vi "TLB Native Dynamic Events ver 0.16.vi"() -> ()   [LabVIEW 2018]
uses:
  Labview Training Phase 2/Enum Controls/States for Action Engine.ctl
  TLB Type Definitions/State Type Definitions.ctl
  TLB Type Definitions/Intruction Type Definitions.ctl
  TLB Type Definitions/Encoder cluster.ctl
  TLB Type Definitions/PING CLUSTER.ctl
  <vilib>/Studica/Studica Toolkit/NavX/NavX.lvlib
  <vilib>/Studica/Studica Toolkit/Background/DIO Channel.ctl
  Underlying VI's/NavX VI/navX type def.ctl
  <vilib>/myRIO/Instrument Drivers/Utilities/Utilities.lvlib
  <vilib>/Studica/Studica Toolkit/Background/I2C Channel.ctl
  TLB Type Definitions/Vision cluster.ctl
  <vilib>/NI_Real-Time Target Support.lvlib
  TLB Type Definitions/Stepper cluster.ctl
  Experimental VI's/Archived VI's/MOTOR CONTROL NO PID Type Def.ctl
  Underlying VI's/I2C Master VI/I2C MASTER Type Def.ctl
  Underlying VI's/I2C Master VI/I2C_MASTER_WRITE_NEW Type Def.ctl
  <vilib>/userdefined/High Color/IMAQdx.ctl
  Underlying VI's/I2C Master VI/Arduino_Interfacing.ctl
  TLB Type Definitions/Yaw Cluster.ctl
  TLB Type Definitions/Time cluster.ctl
  TLB Type Definitions/Y Stepper cluster.ctl
  Underlying VI's/Modified webcam FGV/Webcam AE.ctl
  Underlying VI's/Elasped Timer/Elapsed timer control.ctl
  Underlying VI's/Motor Control VI with PID/MOTOR CONTROL WITH PID AE DATA MODE TYPE DEF.ctl
  Underlying VI's/Motor Control VI with PID/MOTOR CONTROL WITH PID AE DIRECTION TYPE DEF.ctl
  <vilib>/Utility/RT CPU Load.ctl
panel:
  out "Speed & distance":T1
  out "Object Center Coordinates":cluster{"x":sgl, "y":sgl}
  out "Object detection cluster":T2
  out "Time up flag":bool
  out "Task selection":u8
  in  "Object recognition mode":enum16{"Ball", "Soap", "Gel", "Pipe", "None"}(ring)
  out "NavX Readings":T3
  out "Arduino Data":T4
  out "CPU loads":T5[](array[typedef]) {"ISR (%)" format="%#.2f"; "Idle (%)" format="%#.2f"; "Background (%)" format="%#.2f"; "Normal (%)" format="%#.2f"; "Above Normal (%)" format="%#.2f"; "High (%)" format="%#.2g"; "Timed Structures (%)" format="%#.2g"; "Time Critical (%)" format="%#.2g"; "Total (%)" format="%#.2g"}
  out "TASK ENABLE":bool
  out "Rising Edge":bool
  in  "Green LED":bool
  out "Obstacle detected":bool
  out "I2C Error":errorcluster
  out "State Logic":T6=enum."Startup"
  out "elements":T7[](array[typedef])
  in  "STOP TASK":bool
  in  "OK Button":bool
  in  "STOP":bool
  out "error out":errorcluster
  out "Action Queue Items":i32
  out "State Logic Queue Items":i32
  out "Action Queues items":string[](array[string])=["Hardware reset", "Software reset", ""]
  out "Action State":string
  # "System Health Status Update"
  # "VISION"
  # "TLB FRAMEWORK STATUS"
  # "Test Programme written by Calvin Loke    Dated: 28 Aug 2019\nTest Programme revised by Dr Alex See   Dated 30 Aug 2019\n\nRevision date: 20/03/2020\nProgramme version:   TLB Native Dynamic Events ver 0.14a"
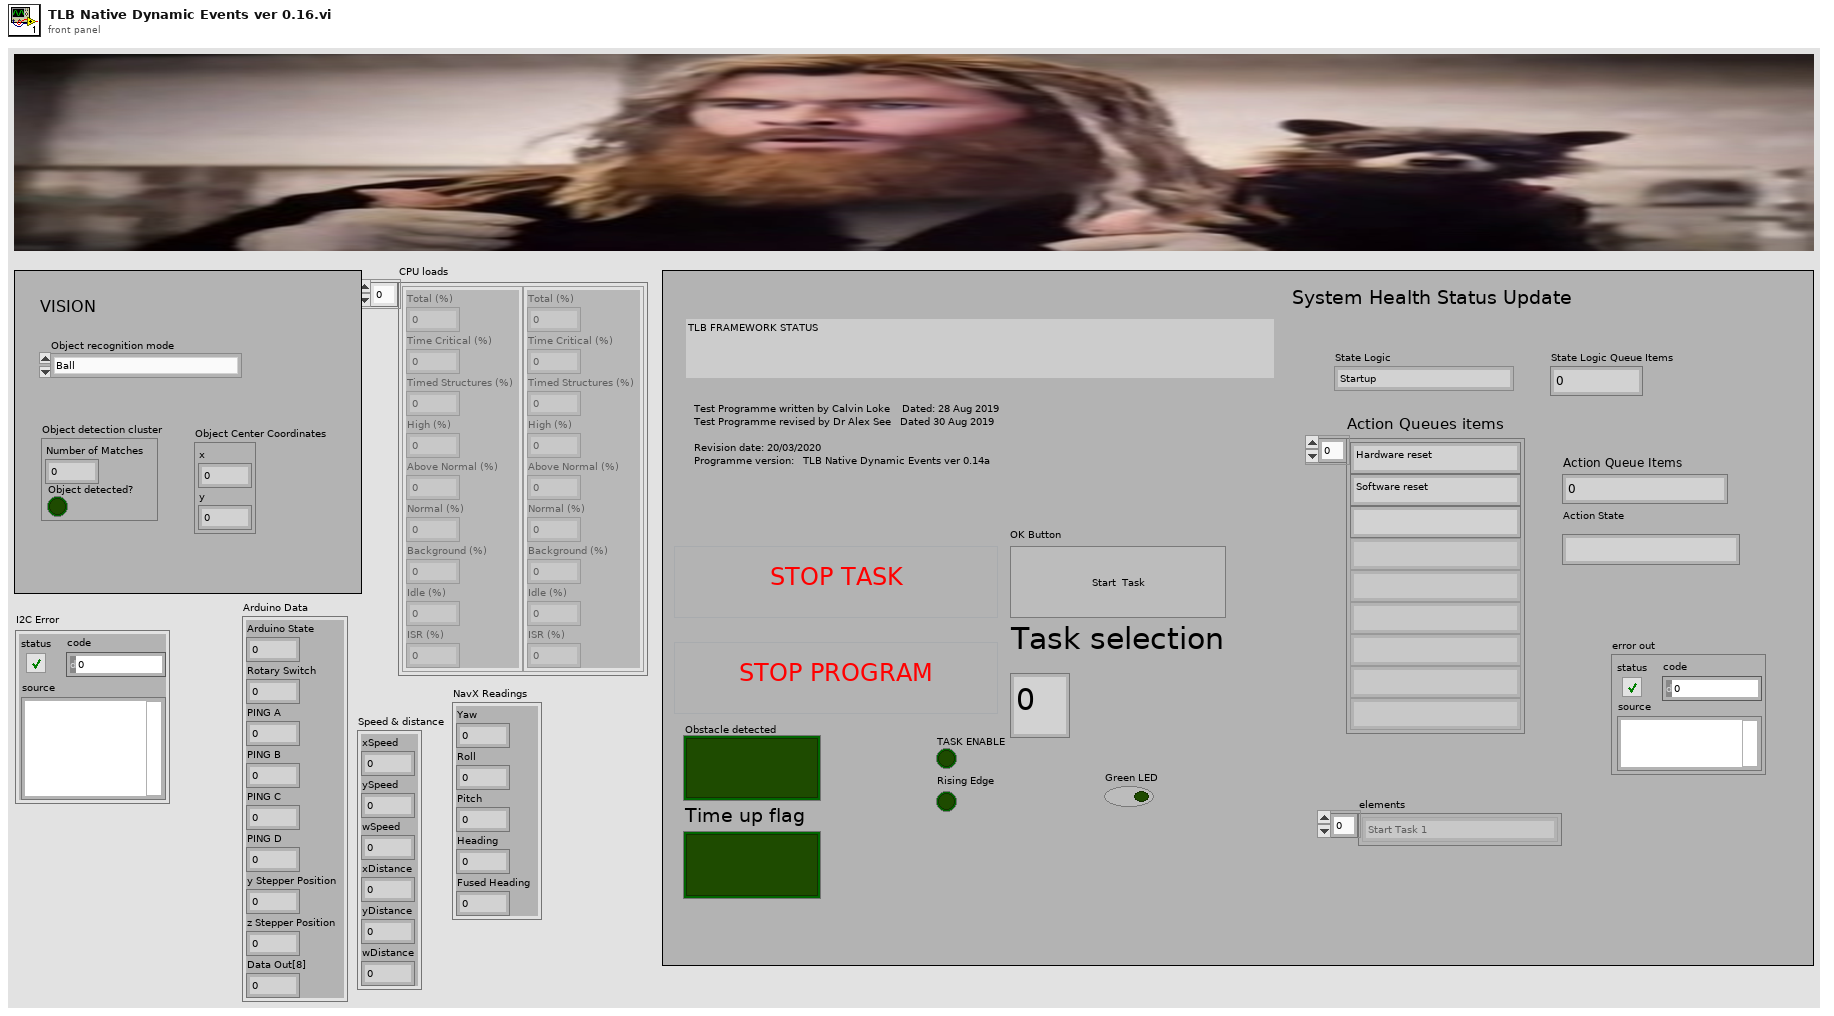
[diagram p1: front panel]
types:
  T1 = cluster{"xSpeed":dbl, "ySpeed":dbl, "wSpeed":dbl, "xDistance":dbl, "yDistance":dbl, "wDistance":dbl}
  T2 = cluster{"Number of Matches":i32, "Object detected?":bool}
  T3 = cluster{"Yaw":dbl, "Roll":dbl, "Pitch":dbl, "Heading":dbl, "Fused Heading":dbl}
  T4 = cluster{"Arduino State":u8, "Rotary Switch":u8, "PING A":u8, "PING B":u8, "PING C":u8, "PING D":u8, "y Stepper Position":u8, "z Stepper Position":u8, "Data Out[8]":u8}
  T5 = typedef "NI_Real-Time Target Support.lvlib/RT CPU Load.ctl" = cluster{"Total (%)":dbl, "Time Critical (%)":dbl, "Timed Structures (%)":dbl, "High (%)":dbl, "Above Normal (%)":dbl, "Normal (%)":dbl, "Background (%)":dbl, "Idle (%)":dbl, "ISR (%)":dbl}
  T6 = typedef "State Type Definitions.ctl" = enum16{"None", "Startup", "Move to Angle", "True Stop", "Idle", "Shutdown", "Task 1A", "Task 1B", "Task 2:Raise Arm", "Task 2:Sensor Mode", "Task 2:Reverse Mode", "Task 3", "Task 4_A", "Task 4_B", "Task 4_C", "Task 4_D", "Task 5A", "Task 5B", "Task 5C", "Task 5D", "Task 5E: POSITION ARM", "Task 5F: ARM GRAB HEIGHT", "Task 5G: CLOSE CLAW", "Task 5H: RAISE ARM", "Task 6_A", "Task 6_B", "Task 7", "Task 8A: RAISE ARM", "Task 8B: MOVE TO BOX", "Task 8C: CAM BURST", "Task 8D: PROCESS IMAGE", "Task 8E: ROBOT ADJUST", "Task 8F: CAM BURST 2", "Task 8G: PROCESS IMAGE 2", "Task 8H: ARM ADJUST", "Task 8I: ARM GRAB HEIGHT", "Task 8J: CLOSE CLAW", "Task 8K: RAISE MY SWORD", "Task 9A: Raise Arm", "Task 9B: Rotate to Angle", "Task 9C: Detect Box", "Task 9D: MOVE FORWARD", "Task 9E: MOVE LEFT", "Task 9F: SCAN IMAGE", "Task 9G: PROCESS COLOUR", "Task 9H: MOVE RIGHT", "Task 9I: SCAN IMAGE", "Task 9J: PROCESS COLOUR", "Task 9K: ROTATE 90 CW", "Task 9L: MOVE FORWARD", "Task 9M: MOVE RIGHT", "Task 9N: SCAN IMAGE", "Task 9O: PROCESS COLOUR", "Task 9P: MOVE RIGHT", "Task 9Q: SCAN IMAGE", "Task 9R: PROCESS COLOUR", "Task A1: Raise Arm", "Task A2: Rotate to Angle", "Task A3: Move Forward", "Task A4: Rotate CW 90"}
  T7 = typedef "Intruction Type Definitions.ctl" = enum16{"None", "Start Task 1", "Start Task 2", "Start Task 3", "Start Task 4", "Start Task 5", "Start Task 6", "Start Task 7", "Start Task 8 - BALL", "Start Task 8 - Gel", "Start Task 8 - Pipe", "Start Task 8 - Soap", "Start Task 9", "Start Task A", "Start Task B", "Exit"}
  T8 = typedef "Y Stepper cluster.ctl" = cluster{"yStepper desired":u8}
  T9 = typedef "Time cluster.ctl" = cluster{"Time up flag":bool, "SET TIME TO CHECK":dbl}
  T10 = typedef "Yaw Cluster.ctl" = cluster{"Yaw":dbl, "Compass":dbl}
  T11 = typedef "Stepper cluster.ctl" = cluster{"y Stepper Position":u8, "z Stepper Position":u8}
  T12 = typedef "DIO Channel.ctl" = enum16{"Not Connected", "A/DIO1", "A/DIO2", "A/DIO3", "A/DIO4", "A/DIO5", "A/DIO6", "A/DIO7", "A/DIO13", "B/DIO1", "B/DIO2", "B/DIO3", "B/DIO4", "B/DIO5", "B/DIO6", "B/DIO7", "B/DIO13", "C/DIO0", "C/DIO1", "C/DIO2", "C/DIO3", "C/DIO4", "C/DIO5", "C/DIO6", "C/DIO7"}
  T13 = typedef "Vision cluster.ctl" = cluster{"Recognized Object":bool, "Object X coordinate":dbl, "Object Y coordinate":dbl}
  T14 = typedef "PING CLUSTER.ctl" = cluster{"PING_A":u8, "PING_B":u8, "PING_C":u8, "PING_D":u8}
  T15 = typedef "Encoder cluster.ctl" = cluster{"xDistance":dbl, "yDistance":dbl, "wDistance":dbl}
  T16 = cluster{"DIO Channel":T12, "FPGA VI Reference Out":refnum<k20>}
  T17 = typedef "navX type def.ctl" = enum16{"Get i2C reference", "Read Values", "Zero Yaw"}
  T18 = typedef "Arduino_Interfacing.ctl" = enum16{"Initialize", "Write to Arduino", "Read From Arduino"}
  T19 = typedef "I2C Channel.ctl" = enum16{"Not Connected", "A", "B"}
  T20 = typedef "States for Action Engine.ctl" = enum16{"Initialize", "Write", "Read"}
  T21 = cluster{"I2C Ref Out":cluster{"I2C Channel":T19, "FPGA VI Reference Out":refnum<k20>}, "Connected":bool, "Slave Address (7-bit)":u8, "Registry":u8[]}
  T22 = typedef "IMAQ Image.ctl" = refnum<image>
  T23 = typedef "State Type Definitions.ctl" = enum16{"None", "Startup", "Move to Angle", "True Stop", "Idle", "Shutdown", "Task 1", "Task 2", "Task 3", "Task 4_A", "Task 4_B", "Task 4_C", "Task 4_D", "Task 5_A", "Task 5 _B", "Task 5_C", "Task 5_D", "Task 5_D_Error", "Task 5D_Error_Right", "Task 5D_Error_Left", "Task 5_E", "Task 5_F", "Task 5F_Error", "Task 5G", "Task 5H", "Task 5I", "Task 6_A", "Task 6_B", "Task 7", "Task 8", "Task 9", "Task A", "Task B"}
  T24 = typedef "MOTOR CONTROL WITH PID AE DIRECTION TYPE DEF.ctl" = enum16{"y-axis movement", "x-axis movement", "rotation", "stop", "reset encoders"}
  T25 = typedef "MOTOR CONTROL WITH PID AE DATA MODE TYPE DEF.ctl" = enum16{"Init AE", "Write to AE", "Read from AE"}
  T26 = typedef "Elapsed timer control.ctl" = enum16{"Start", "Pause", "Initialize"}
  T27 = typedef "I2C_MASTER_WRITE_NEW Type Def.ctl" = enum16{"Ultrasonic sensors", "Stepper origin", "zStepper 13.3k", "zStepper 13k", "zStepper 12k", "zStepper 11k", "zStepper 10k", "zStepper 9k", "zStepper 8k", "zStepper 7k", "zStepper 6k", "zStepper 5k", "zStepper 4k", "zStepper 3k", "zStepper 2k", "zStepper 1k", "zStepper 900", "zStepper 800", "zStepper 700", "zStepper 600", "zStepper 500", "zStepper 400", "zStepper 300", "zStepper 200", "zStepper 100", "zStepper 0", "yStepper control", "Open Claw", "Close Claw", "Soft Reset"}
  T28 = typedef "Webcam AE.ctl" = enum16{"Initialize Camera", "Open Camera", "Continuous Acquisition", "Close Camera", "Retrieve Image", "Dispose Camera Image Buffer"}
  T29 = typedef "IMAQdx.ctl" = refnum<k21>
  T30 = typedef "Webcam AE.ctl" = enum16{"Initialize Camera", "Open Camera", "Continuous Acquisition", "Close Camera", "Retrieve Image", "Dispose Image Buffers"}
  T31 = typedef "MOTOR CONTROL NO PID Type Def.ctl" = enum16{"Init", "Front Back", "Left Right", "Rotate", "Stop", "Latch"}
  T32 = typedef "I2C MASTER Type Def.ctl" = enum16{"Last State", "Mode 0", "Mode 1", "Mode 2", "Mode 3", "Mode 4", "Mode 5", "Mode 6", "Mode 7", "Mode 8", "Mode 9", "Mode 10"}
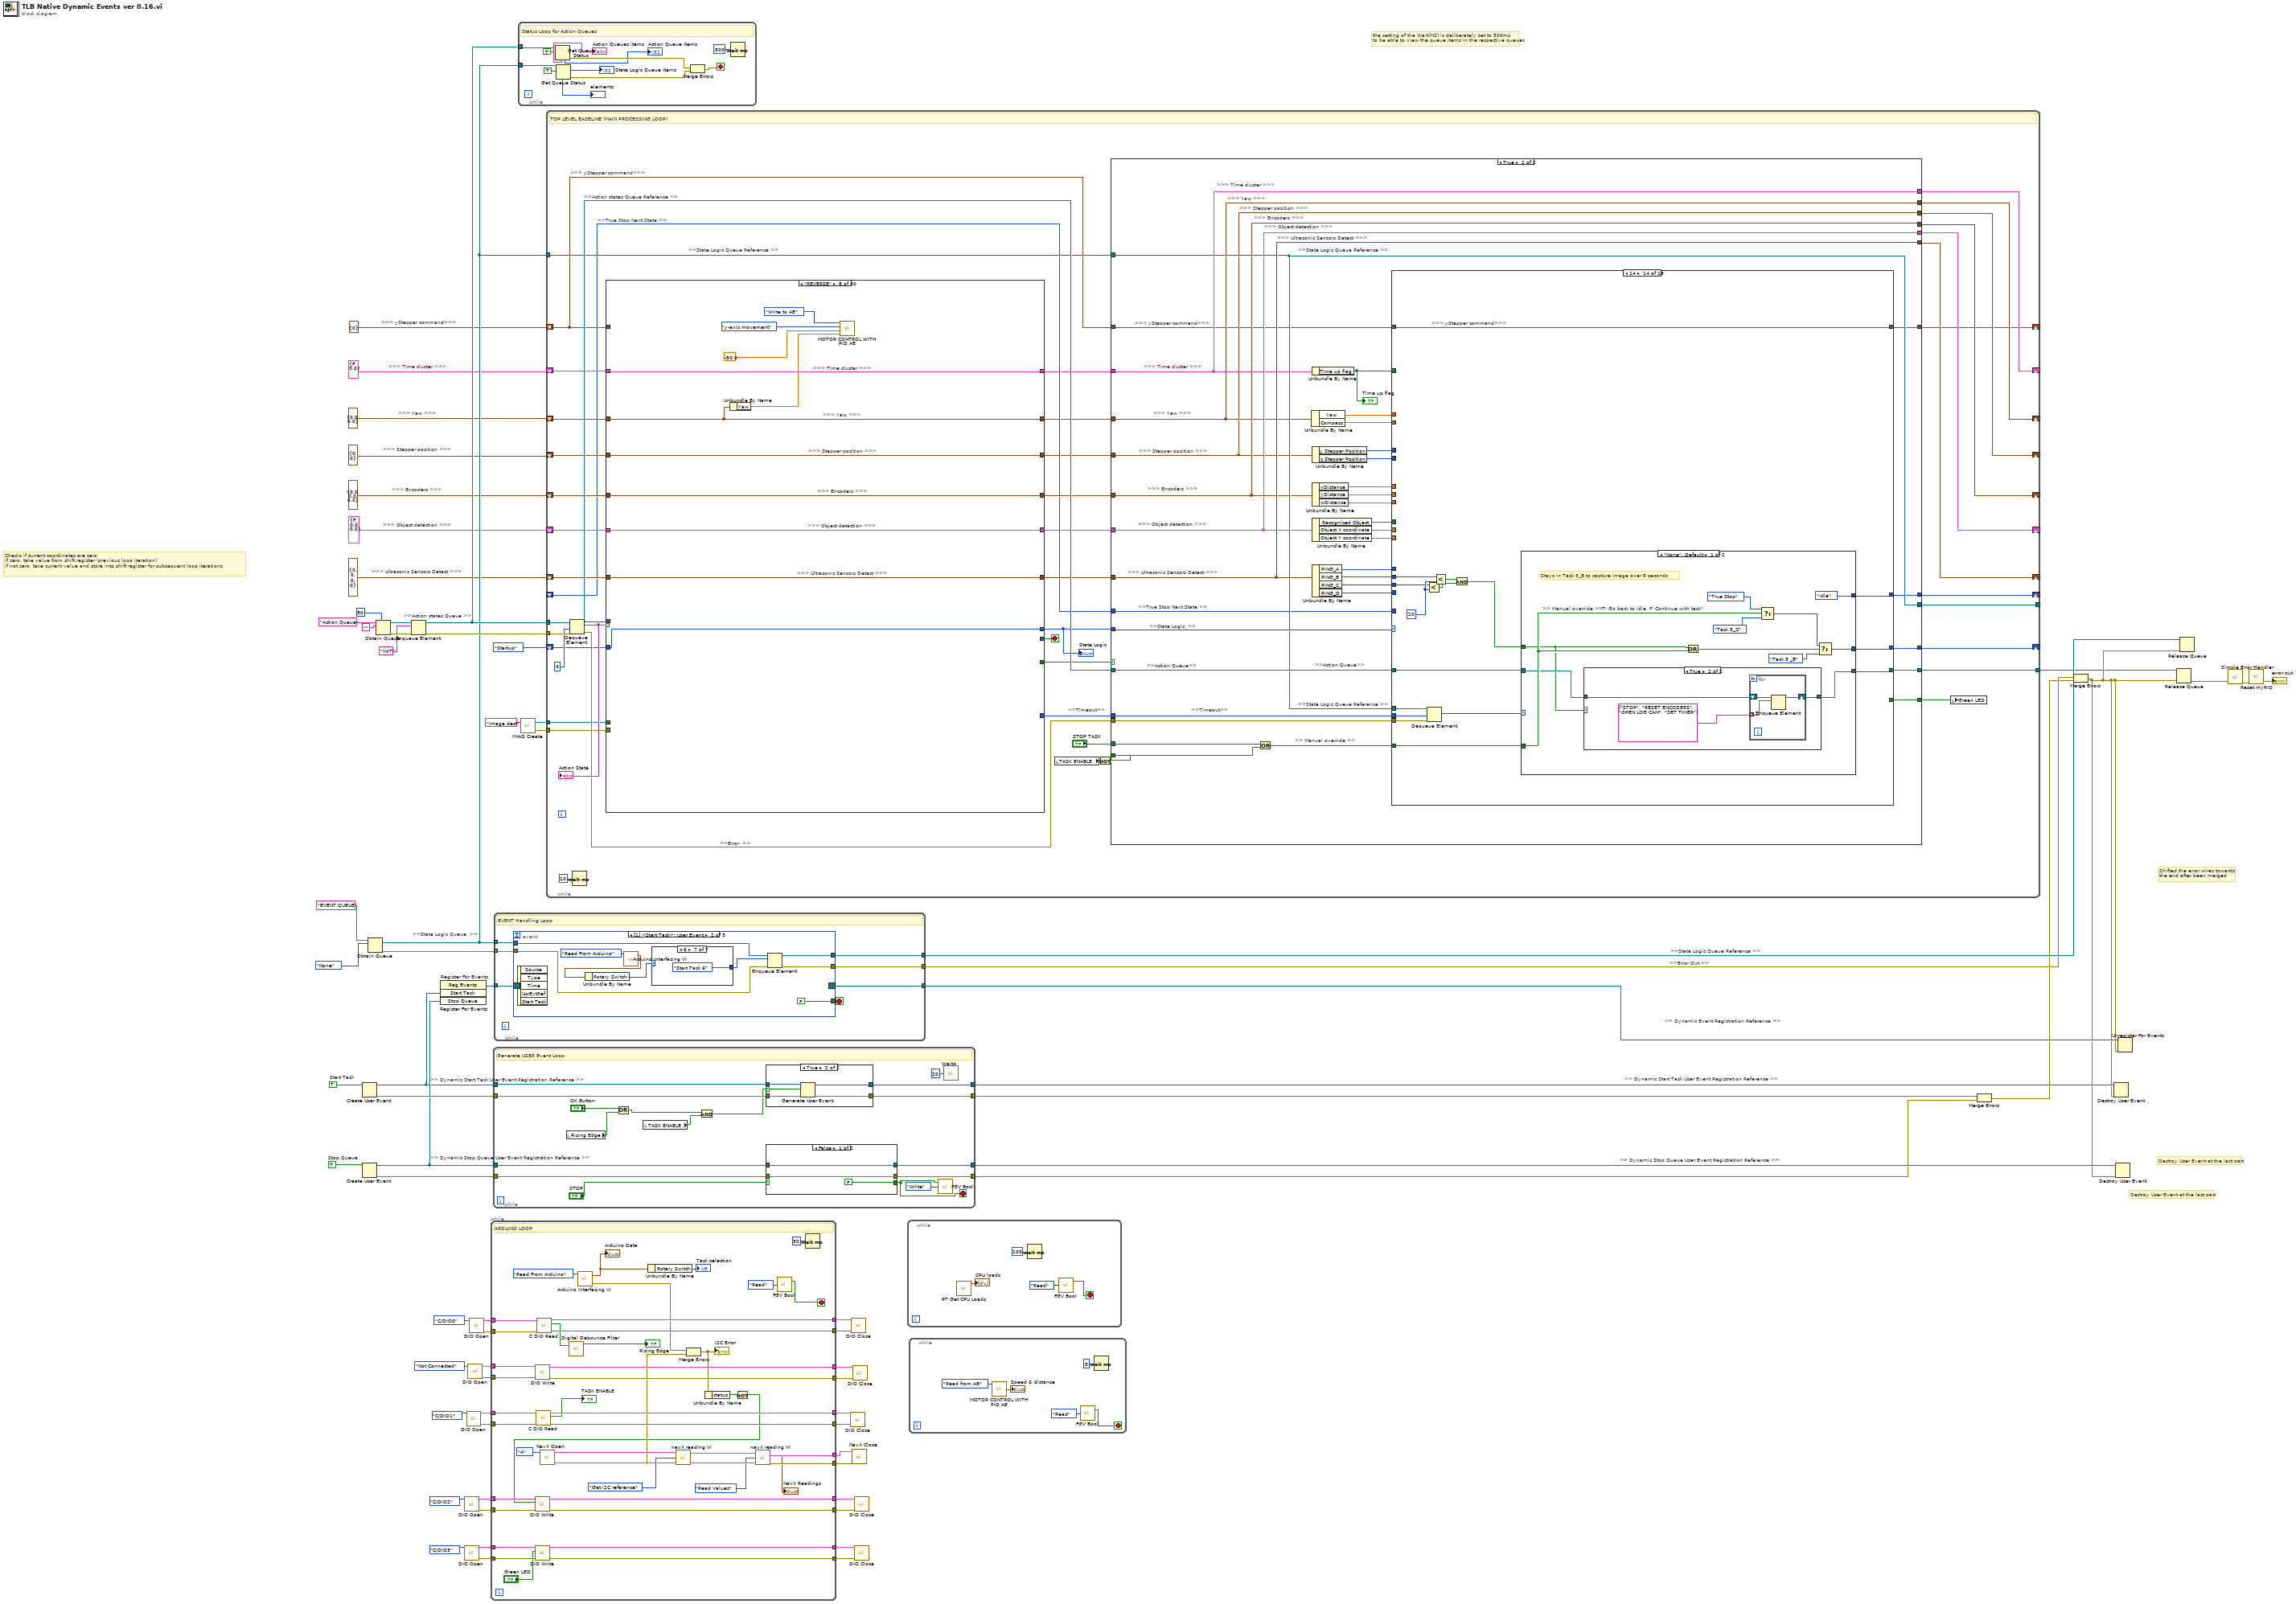
[diagram p0: block diagram]
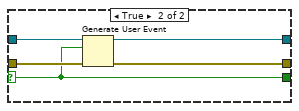
[diagram p2: hidden frame]
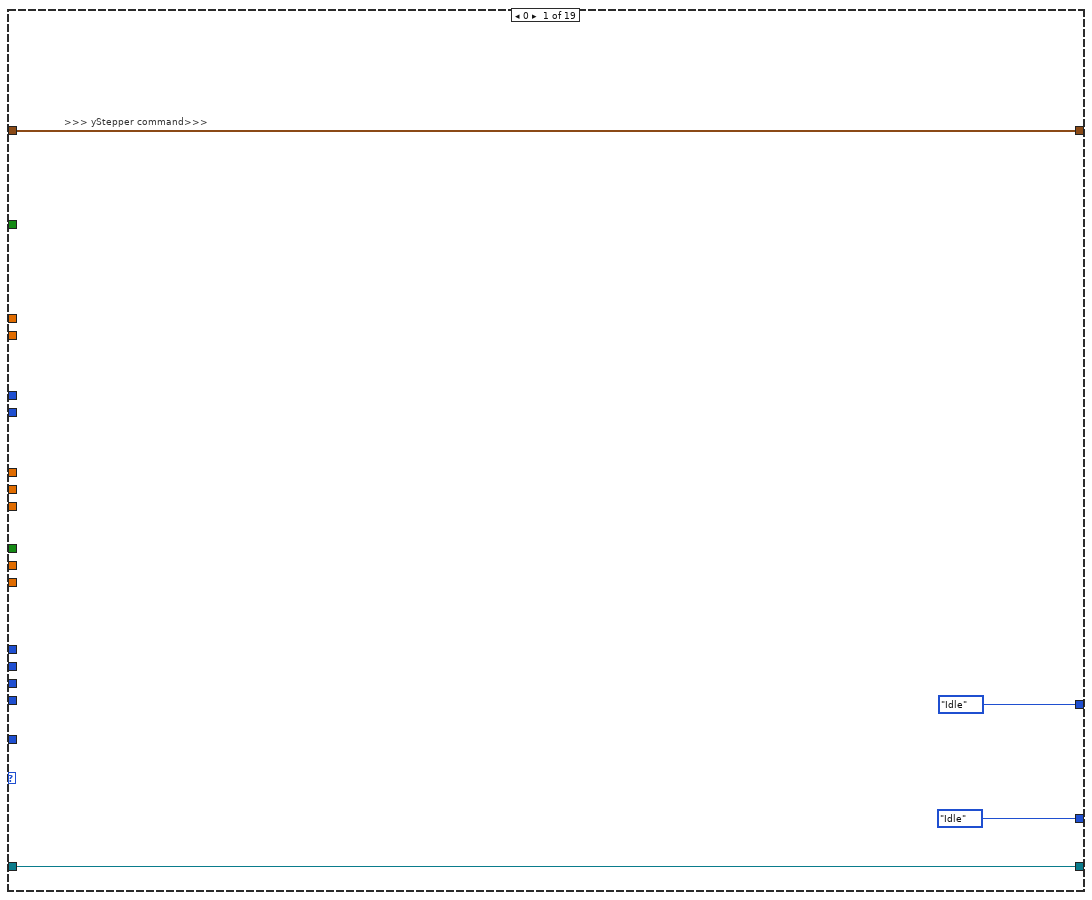
[diagram p5: hidden frame]
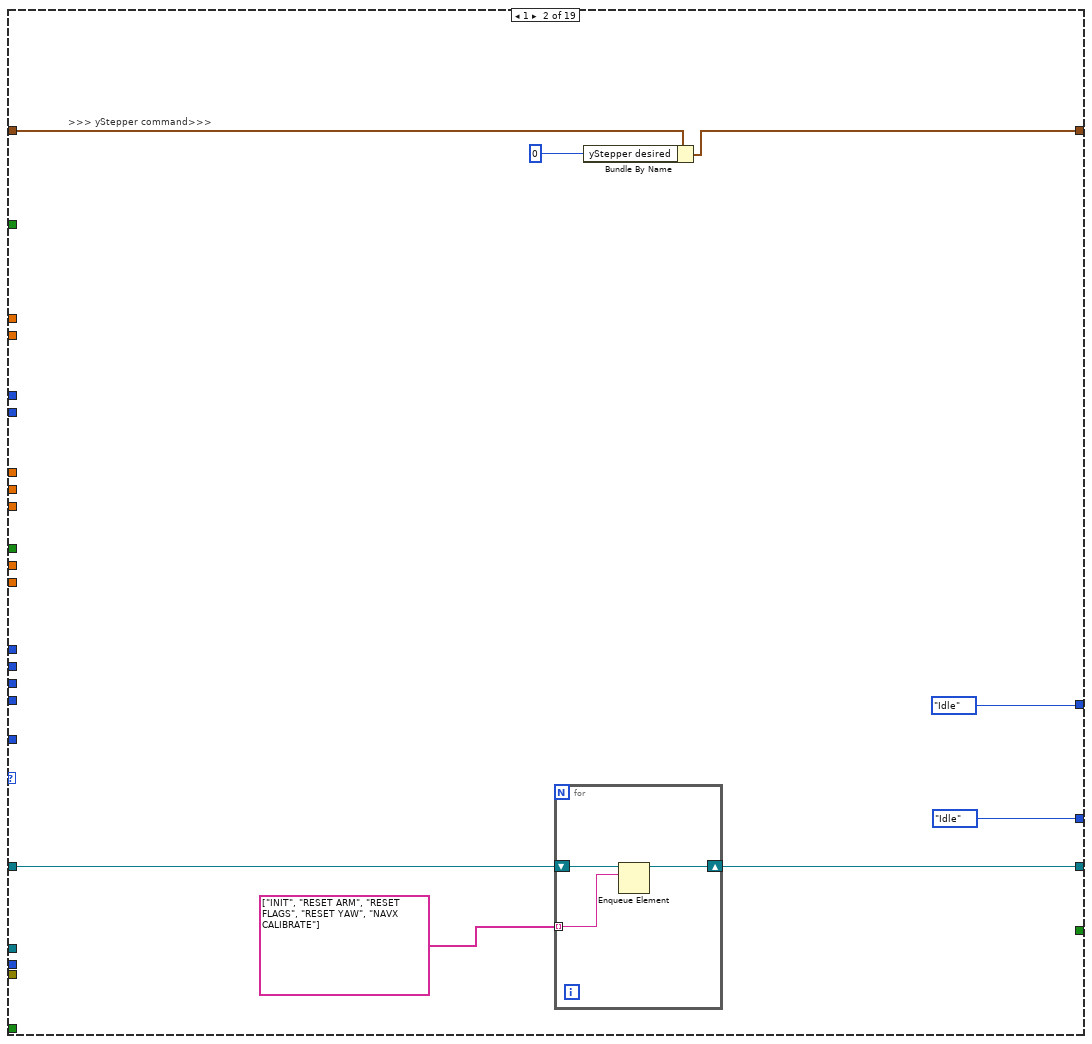
[diagram p6: hidden frame]
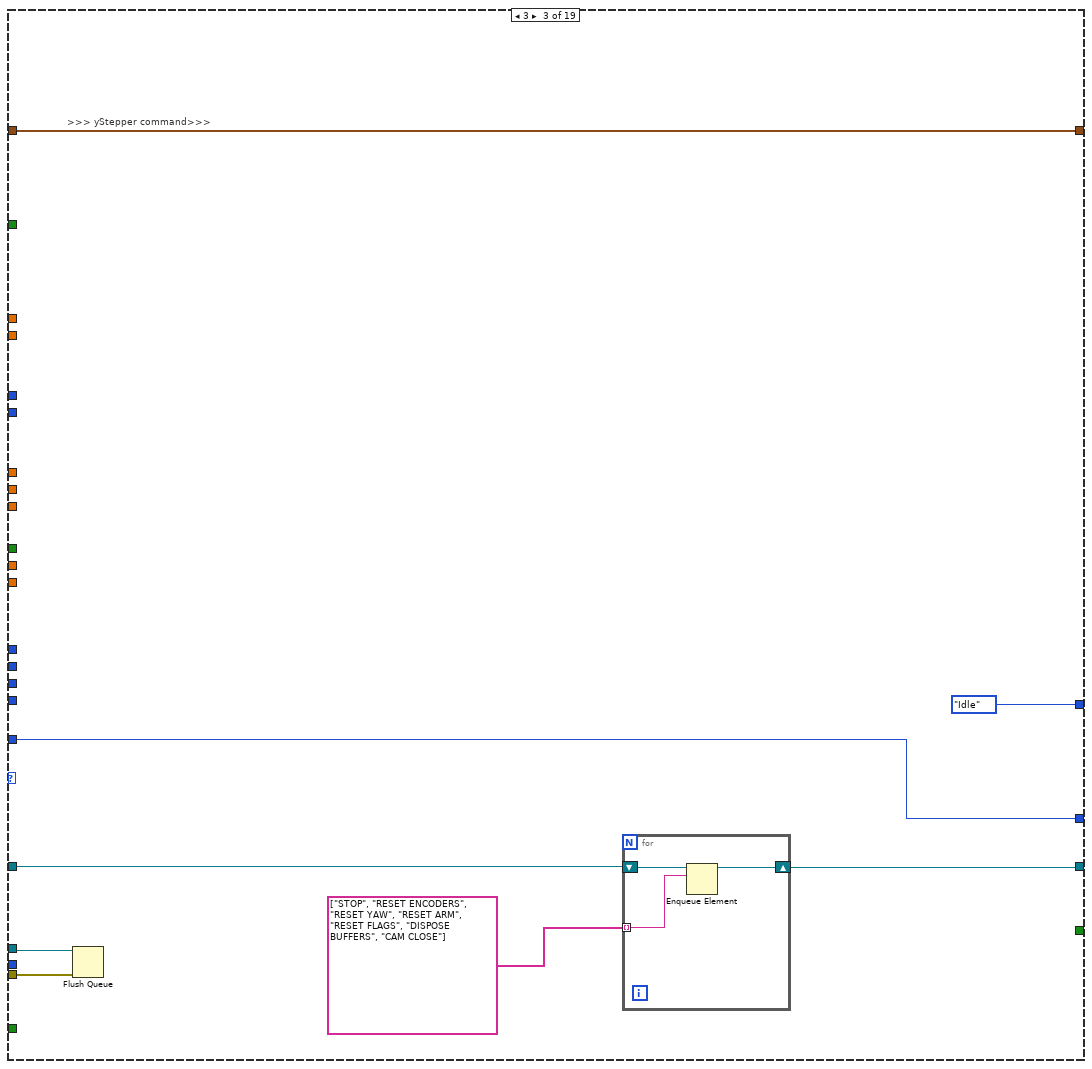
[diagram p7: hidden frame]
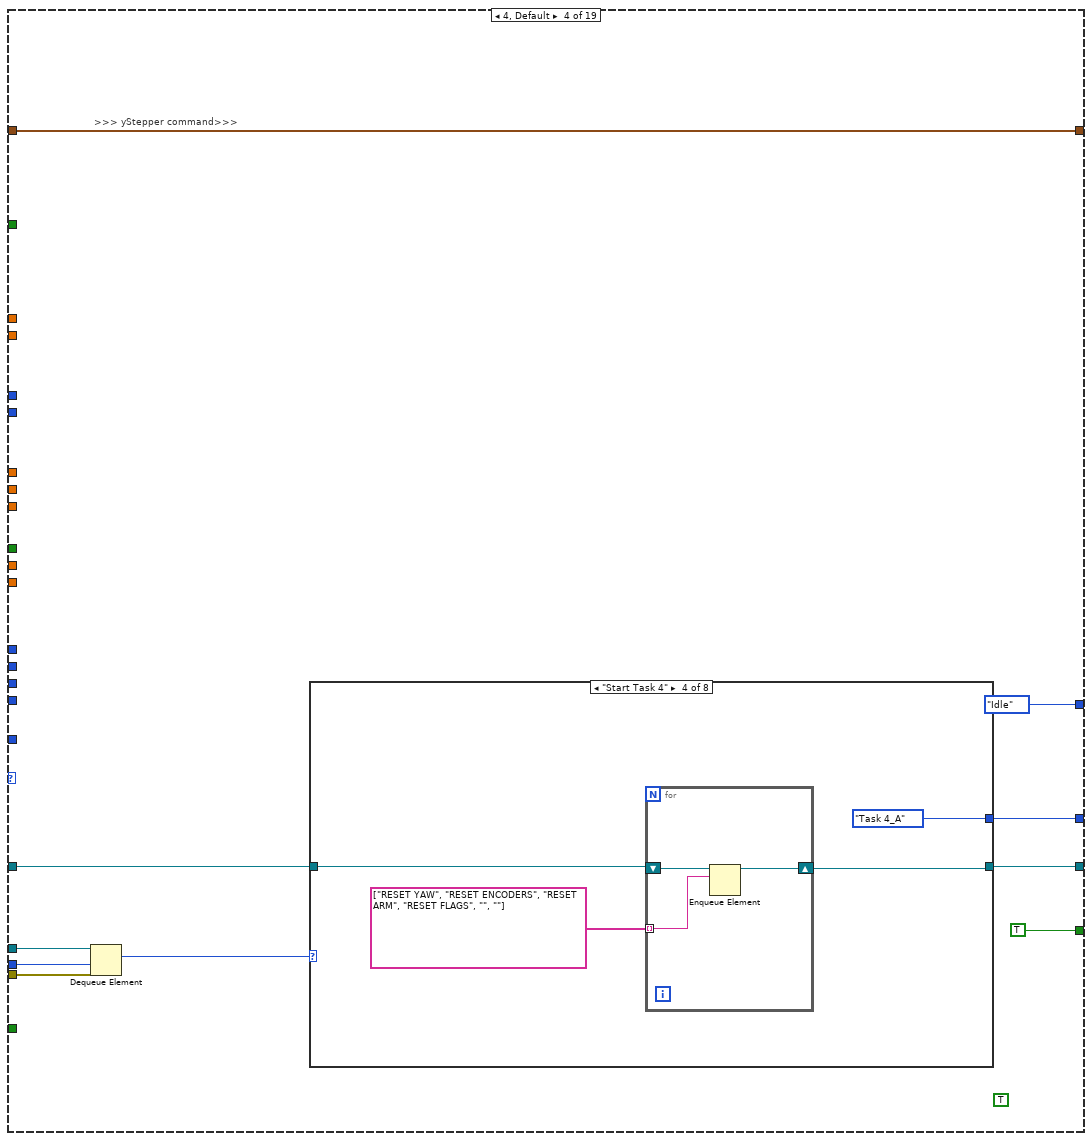
[diagram p8: hidden frame]
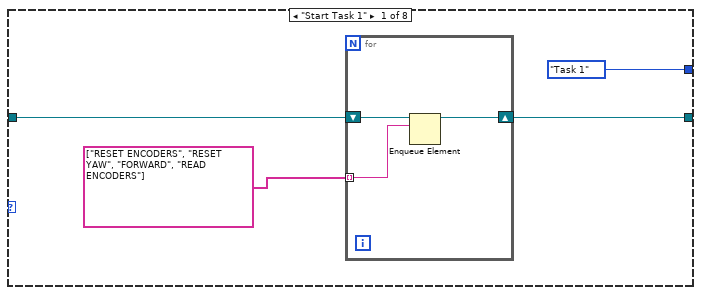
[diagram p9: hidden frame]
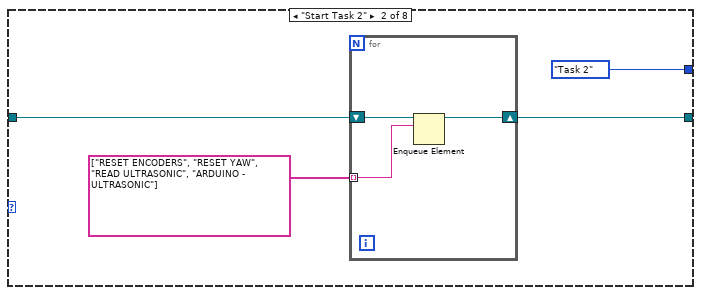
[diagram p10: hidden frame]
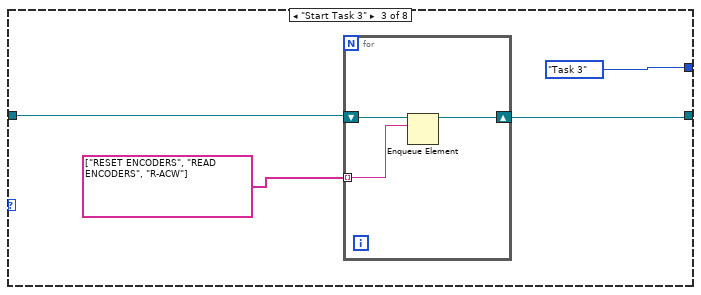
[diagram p11: hidden frame]
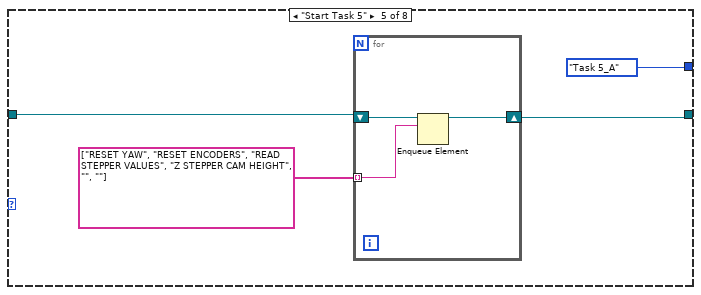
[diagram p12: hidden frame]
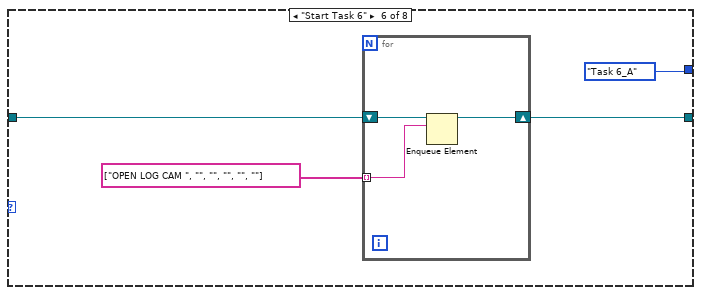
[diagram p13: hidden frame]
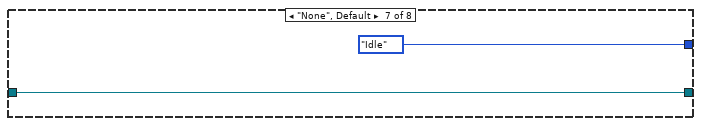
[diagram p14: hidden frame]
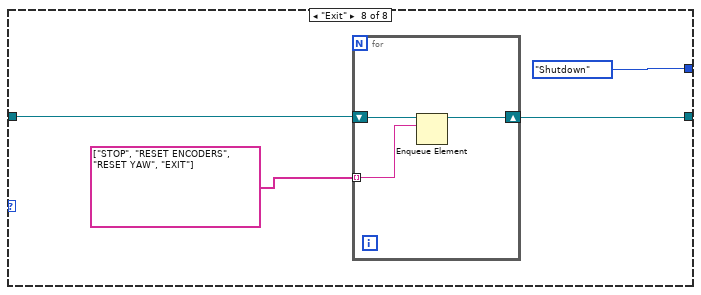
[diagram p15: hidden frame]
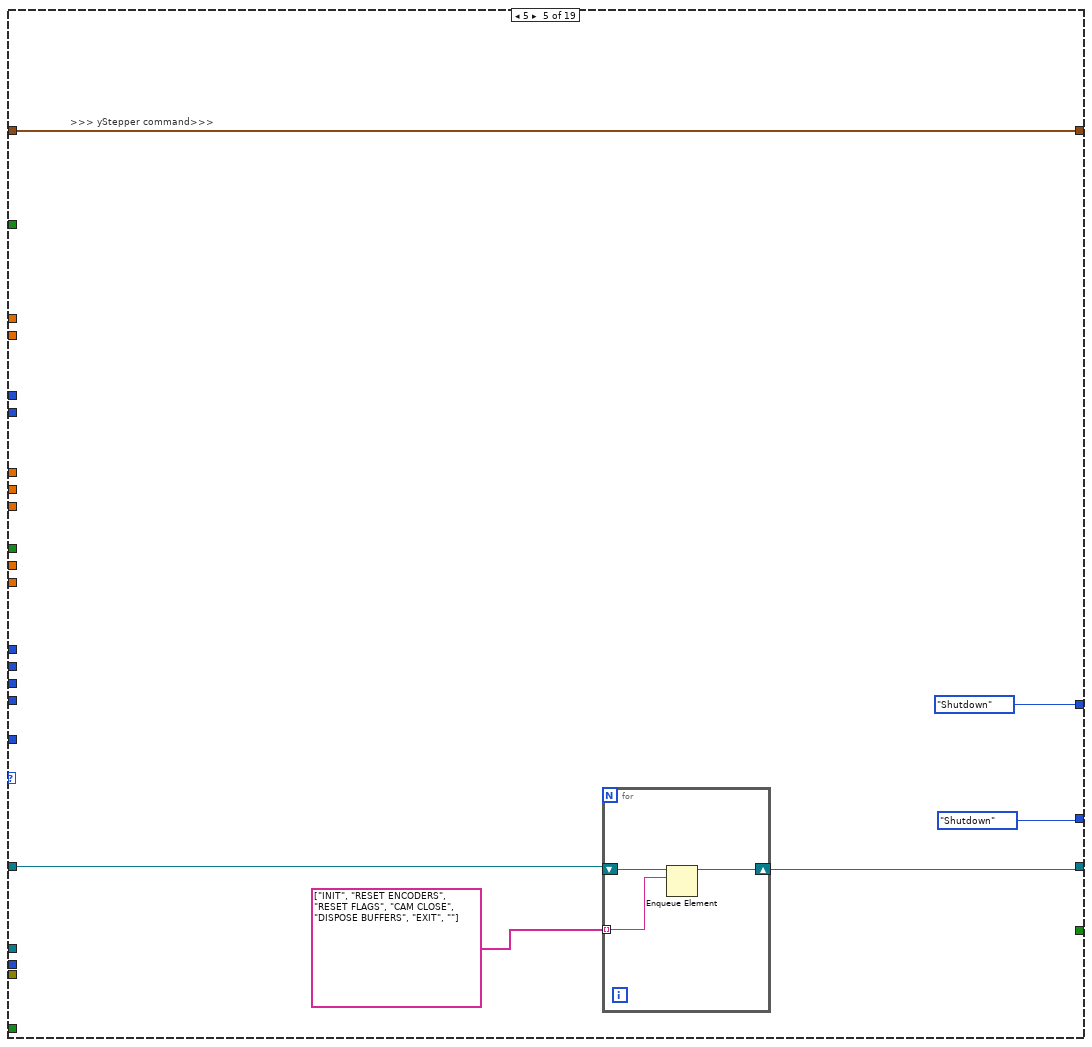
[diagram p16: hidden frame]
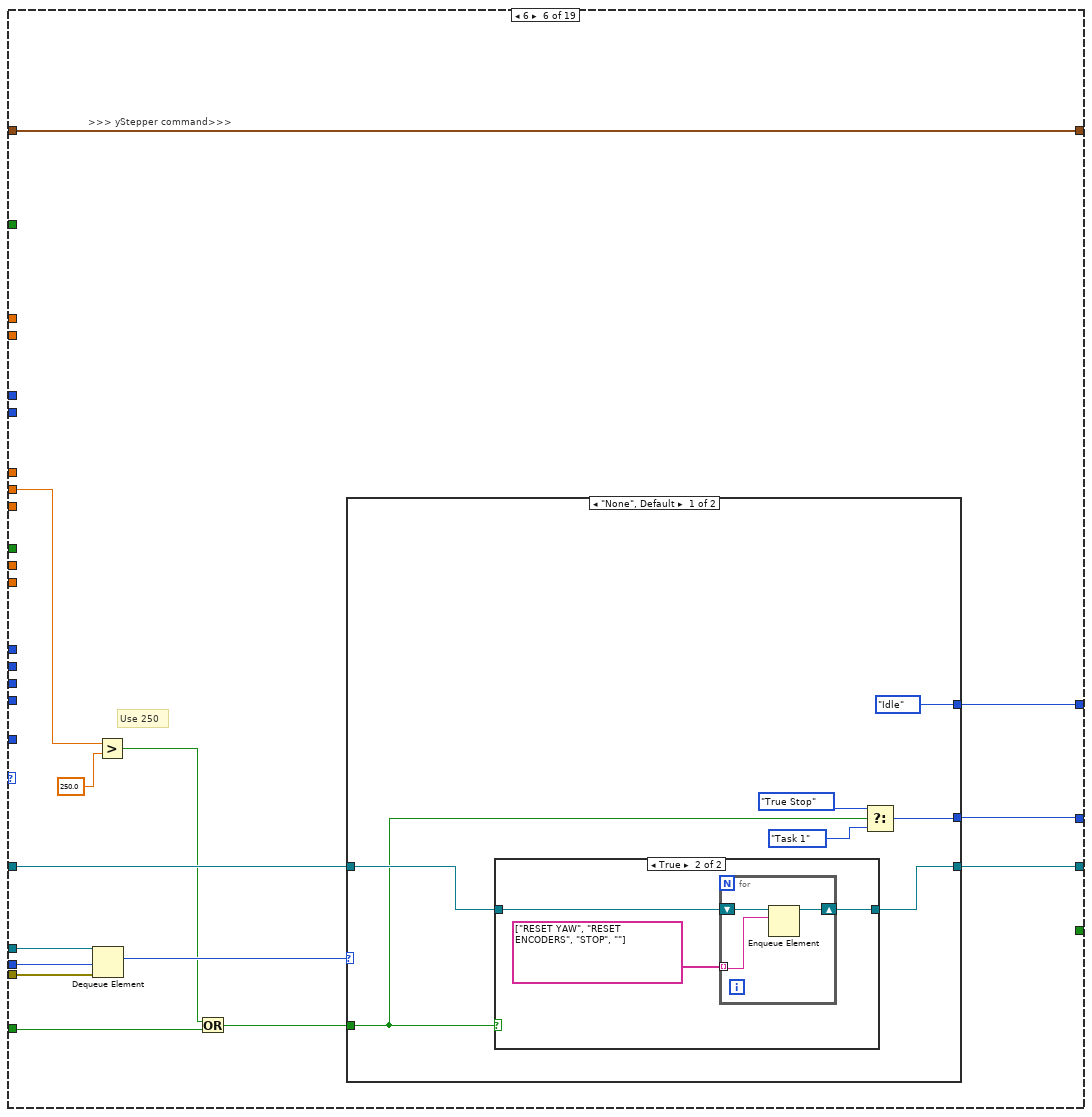
[diagram p17: hidden frame]
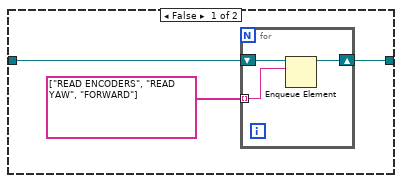
[diagram p18: hidden frame]
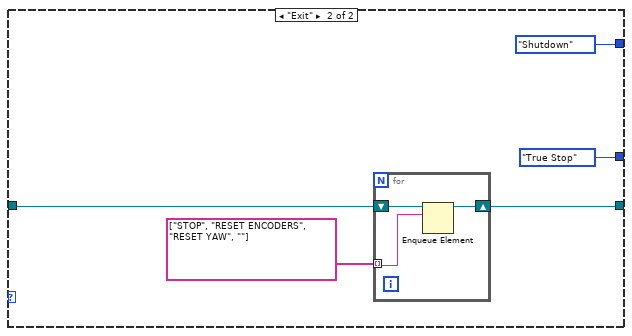
[diagram p19: hidden frame]
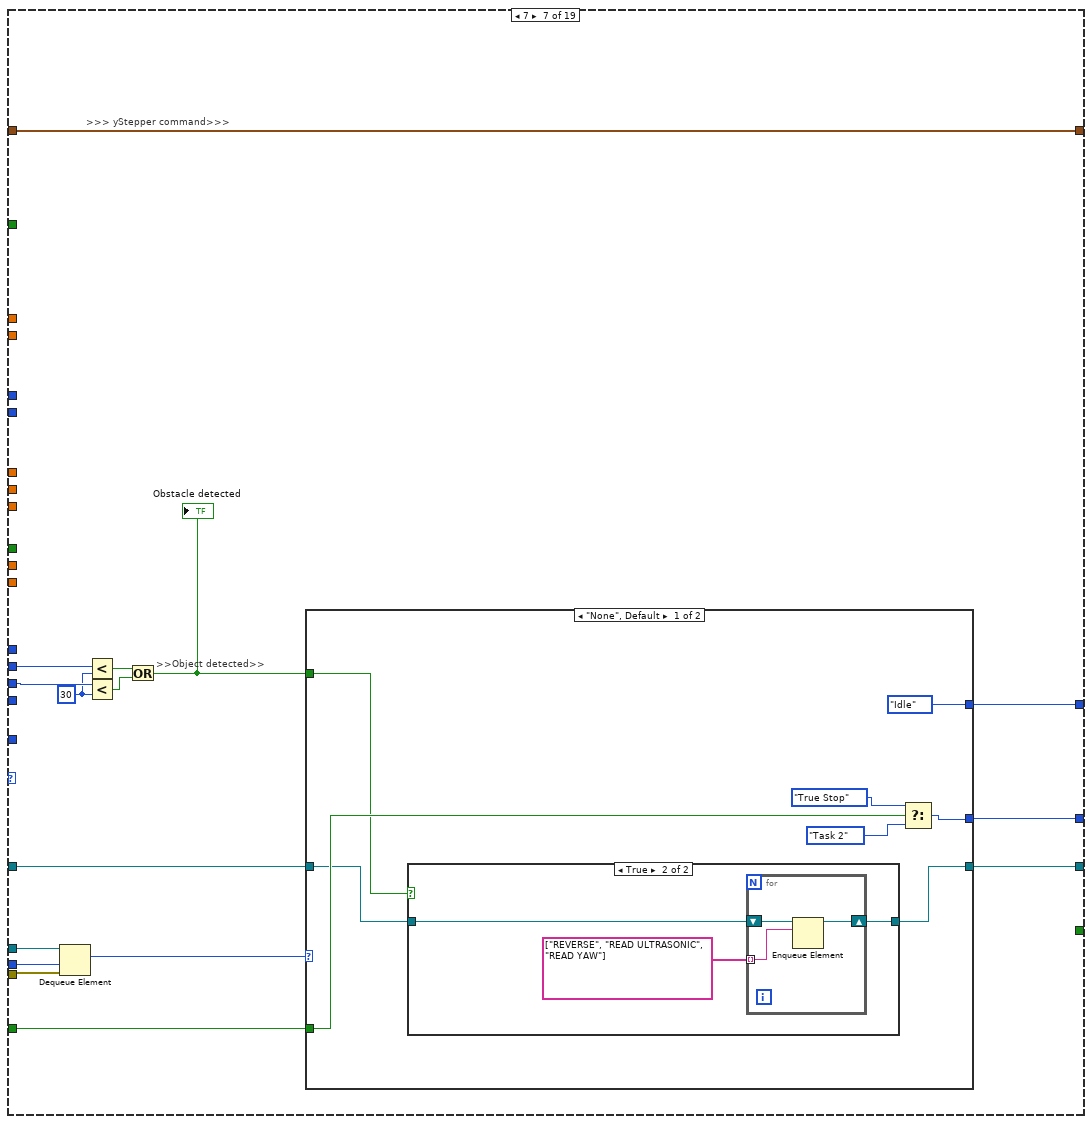
[diagram p20: hidden frame]
diagram:
  w70 = TRUE  # Stop Queue
  w69 = TRUE  # Start Task
  # "Checks if current coordinates are zero\nif zero, take value from shift register (previous loop iteration)\nif not zero, take current value and store into shift register for subsequent loop iterations"
  # ">>> yStepper command>>>"
  # ">>> Time cluster >>>"
  # ">>> Yaw >>>"
  # ">>> Stepper position >>>"
  # ">>> Encoders >>>"
  # ">>> Object detection >>>"
  # ">>> Ultrasonic Sensors Detect >>>"
  # "the setting of the Wait(MS) is deliberately set to 500ms\nto be able to view the queue items in the respective queues"
  # ">>Error Out >>"
  # ">> Dynamic Stop Queue User Event Registration Reference >>"
  # ">> Dynamic Start Task User Event Registration Reference >>"
  # ">> Dynamic Stop Queue User Event Registration Reference >>"
  # ">> Dynamic Start Task User Event Registration Reference >>"
  # ">> Dynamic Event Registration Reference >>"
  # ">>Action states Queue >>"
  # ">>State Logic Queue  >>"
  # ">>State Logic Queue Reference >>"
  # "Destroy User Event at the last part"
  # "Destroy User Event at the last part"
  # "Shifted the error wires towards\nthe end after been merged"
  n1 = Create User Event(user event datatype=w69) -> (user event=w61:refnum<user-event>, error out=w66:errorcluster)  [unwired: 1 in]
  n2 = Create User Event(user event datatype=w70) -> (user event=w62:refnum<user-event>, error out=w65:errorcluster)  [unwired: 1 in]
  n3 = Obtain Queue(name (unnamed)="EVENT QUEUE", element data type=Intruction_Type_Definitions."None" ("Enum")) -> (queue out=w47:refnum<queue>, error out=w53:errorcluster)  [unwired: 3 in, 1 out]
  n4 = Obtain Queue(max queue size (-1, unlimited)=50, name (unnamed)="Action Queue", element data type="") -> (queue out=w56:refnum<queue>, error out=w52:errorcluster)  [unwired: 2 in, 1 out]
  n5 = Enqueue Element(queue=w56, element="INIT", error in (no error)=w52) -> (queue out=w48:refnum<queue>, error out=w51:errorcluster)  [unwired: 1 in, 1 out]
  n6 = register-events "Register For Events"(w61, w62) -> (reference out=w60:refnum<event-registration>)  [unwired: 2 in, 1 out]
  n7 = call <vilib>:"DIO Open.vi"("DIO Channel"=DIO_Channel."C/DIO2") -> ("error out"=w14:errorcluster, "DIO Info Out"=w15:T16)  [unwired: 9 in]
  n8 = call <vilib>:"DIO Open.vi"("DIO Channel"=DIO_Channel."C/DIO3") -> ("error out"=w9:errorcluster, "DIO Info Out"=w10:T16)  [unwired: 9 in]
  n9 = call <vilib>:"DIO Open.vi"("DIO Channel"=DIO_Channel."C/DIO1") -> ("error out"=w25:errorcluster, "DIO Info Out"=w26:T16)  [unwired: 9 in]
  n10 = call <vilib>:"DIO Open.vi"("DIO Channel"=DIO_Channel."Not Connected") -> ("error out"=w30:errorcluster, "DIO Info Out"=w32:T16)  [unwired: 9 in]
  n11 = call <vilib>:"DIO Open.vi"("DIO Channel"=DIO_Channel."C/DIO0") -> ("error out"=w35:errorcluster, "DIO Info Out"=w38:T16)  [unwired: 9 in]
  n12 = while {
    tunnel: w38 -> [w111]
    tunnel: [w110] -> w36
    tunnel: w35 -> [w109]
    tunnel: [w108] -> w34
    tunnel: w32 -> [w105]
    tunnel: [w104] -> w31
    tunnel: w30 -> [w103]
    tunnel: [w102] -> w29
    tunnel: [w101] -> w27
    tunnel: w26 -> [w100]
    tunnel: w25 -> [w99]
    tunnel: [w98] -> w24
    tunnel: w15 -> [w92]
    tunnel: w14 -> [w91]
    tunnel: [w90] -> w13
    tunnel: [w89] -> w12
    tunnel: w10 -> [w88]
    tunnel: w9 -> [w87]
    tunnel: [w86] -> w8
    tunnel: [w85] -> w7
    tunnel: [w79] -> w4
    tunnel: [w78] -> w5
    stop <- w113 stop-if-true
    # "ARDUINO LOOP"
    n13 = call <vilib>:"DIO Write.vi"("error in (no error)"=w87, "Input"="Green LED", "DIO Info In"=w88) -> ("error out"=w85:errorcluster, "DIO Info Out"=w86:T16)  [unwired: 7 in]
    n14 = call <vilib>:"DIO Write.vi"("error in (no error)"=w103, "DIO Info In"=w105) -> ("error out"=w102:errorcluster, "DIO Info Out"=w104:T16)  [unwired: 8 in]
    n15 = call <vilib>:"C DIO Read.vi"("error in (no error)"=w99, "DIO Info In in"=w100) -> ("error out"=w98:errorcluster, "IN"=→"TASK ENABLE":bool, "DIO Info In out"=w101:T16)  [unwired: 7 in]
    n16 = call <vilib>:"C DIO Read.vi"("error in (no error)"=w109, "DIO Info In in"=w111) -> ("error out"=w108:errorcluster, "IN"=w107:bool, "DIO Info In out"=w110:T16)  [unwired: 7 in]
    n17 = call <vilib>:"NavX Open.vi"("I2C Channel"=I2C_Channel."A") -> ("error out"=w94:errorcluster, "NavX Info"=w96:T21)  [unwired: 9 in]
    n18 = call "Digital Debounce Filter.vi"("Boolean input"=w107) -> ("Rising Edge"=→"Rising Edge":bool)  [unwired: 1 in, 2 out]
    n19 = call "Arduino Interfacing VI.vi"("AE Mode"=Arduino_Interfacing."Read From Arduino") -> ("error out"=w82:errorcluster, "Arduino Data"=w75:T4)  [unwired: 3 in]
    "Arduino Data" <- w75
    n20 = Unbundle By Name(w75) -> ("Rotary Switch"=→"Task selection":u8)
    n21 = call "navX reading VI.vi"("NavX Info In"=w96, "Mode"=navX_type_def."Get i2C reference", "error in (no error)"=w94) -> ("NavX Info Out"=w81:T21, "Error Out"=w80:errorcluster)  [unwired: 2 out]
    n22 = Merge Errors(w82, w94) -> (w73:errorcluster)
    "I2C Error" <- w73
    n23 = Unbundle By Name(w73) -> ("status"=w72:bool)
    n24 = Not(x=w72) -> (.not. x?=w71:bool)
    n25 = call <vilib>:"DIO Write.vi"("error in (no error)"=w91, "Input"=w71, "DIO Info In"=w92) -> ("error out"=w89:errorcluster, "DIO Info Out"=w90:T16)  [unwired: 7 in]
    n26 = call "navX reading VI.vi"("NavX Info In"=w81, "Mode"=navX_type_def."Read Values", "error in (no error)"=w80) -> ("NavX Info Out"=w79:T21, "NavX Readings"=→"NavX Readings":T3, "Error Out"=w78:errorcluster)  [unwired: 1 out]
    n27 = call "FGV Bool.vi"("Init/Read/Write State"=States_for_Action_Engine."Read") -> ("Output node"=w113:bool)  [unwired: 2 in, 1 out]
    n28 = Wait (ms)(milliseconds to wait=u32 50) -> ()  [unwired: 1 out]
  }
  n29 = while {
    tunnel: w61 -> [w131]
    tunnel: w62 -> [w130]
    tunnel: [w129] -> w68
    tunnel: [w128] -> w67
    tunnel: w66 -> [w127]
    tunnel: [w126] -> w64
    tunnel: w65 -> [w125]
    tunnel: [w124] -> w63
    stop <- w122 stop-if-true
    # "Generate USER Event Loop"
    n30 = local read "Rising Edge"() -> (w118:bool)
    n31 = Or(x="OK Button", y=w118) -> (x .or. y?=w117:bool)
    n32 = local read "TASK ENABLE"() -> (w116:bool)
    n33 = And(x=w117, y=w116) -> (x .and. y?=w115:bool)
    n34 = case shown="True" w115 {
      selector: w115 -> [_ w142]
      tunnel: w131 -> [w141 w146]
      tunnel: [w141 w145] -> w128
      tunnel: w127 -> [w140 w144]
      tunnel: [w140 w143] -> w126
      frame False {
      }
      frame True {
        n35 = Generate User Event(user event=w146, event data cluster=w142, error in=w144) -> (user event out=w145:refnum<user-event>, error out=w143:errorcluster)  [unwired: 1 in]
      }
    }
    n36 = case shown="False" "STOP" {
      selector: "STOP" -> [_ w135]
      tunnel: w130 -> [w134 w139]
      tunnel: [w134 w138] -> w129
      tunnel: w125 -> [w133 w137]
      tunnel: [w133 w136] -> w124
      tunnel: [FALSE w135] -> w122
      frame False {
      }
      frame True {
        n37 = Generate User Event(user event=w139, event data cluster=w135, error in=w137) -> (user event out=w138:refnum<user-event>, error out=w136:errorcluster)  [unwired: 1 in]
      }
    }
    n38 = call "FGV Bool.vi"("Init/Read/Write State"=States_for_Action_Engine."Write", "Input Node"=w122) -> ()  [unwired: 1 in, 2 out]
    n39 = call "Wait4"("Count(uSec)"=u32 20) -> ()  [unwired: 1 out]
  }
  n40 = while {
    tunnel: w60 -> [w153]
    tunnel: [w152] -> w59
    tunnel: w47 -> [w150]
    tunnel: [w149] -> w58
    tunnel: w53 -> [w148]
    tunnel: [w147] -> w50
    stop <- w151 stop-if-true
    # "EVENT Handling Loop"
    n41 = event shown="[1] <Start Task>: User Event" {
      selector: w153 -> [_ _ _]
      dyn-events: [_ _ _] -> w152
      timeout: _ -> [_ _ _]
      tunnel: [FALSE FALSE w181] -> w151
      tunnel: w150 -> [w158 w167 w179]
      tunnel: [w157 w166 w180] -> w149
      tunnel: w148 -> [w156 w165 w178]
      tunnel: [w155 w164 w177] -> w147
      event Timeout {
        n42 = event-data() -> ()  [unwired: 1 in, 3 out]
        n43 = Enqueue Element(queue=w158, element=Intruction_Type_Definitions."None" ("Enum"), error in (no error)=w156) -> (queue out=w157:refnum<queue>, error out=w155:errorcluster)  [unwired: 1 in, 1 out]
      }
      event User Event {
        n44 = event-data() -> ()  [unwired: 1 in, 5 out]
        n45 = call "Arduino Interfacing VI.vi"("AE Mode"=Arduino_Interfacing."Read From Arduino") -> ("Arduino Data"=w161:T4)  [unwired: 3 in, 1 out]
        n46 = Unbundle By Name(w161) -> ("Rotary Switch"=w160:u8)
        n47 = case shown="6" w160 {
          tunnel: [Intruction_Type_Definitions."None" ("Enum") Intruction_Type_Definitions."Start Task 1" ("Enum") Intruction_Type_Definitions."Start Task 2" ("Enum") Intruction_Type_Definitions."Start Task 3" ("Enum") Intruction_Type_Definitions."Start Task 4" ("Enum") Intruction_Type_Definitions."Start Task 5" ("Enum") Intruction_Type_Definitions."Start Task 6" ("Enum")] -> w163
          frame 0, Default {
          }
          frame 1 {
          }
          frame 2 {
          }
          frame 3 {
          }
          frame 4 {
          }
          frame 5 {
          }
          frame 6 {
          }
        }
        n48 = Enqueue Element(queue=w167, element=w163, error in (no error)=w165) -> (queue out=w166:refnum<queue>, error out=w164:errorcluster)  [unwired: 1 in, 1 out]
      }
      event User Event {
        n49 = event-data() -> ("Stop Queue"=w181:bool)  [unwired: 1 in, 4 out]
        n50 = Enqueue Element At Opposite End(queue=w179, element=Intruction_Type_Definitions."Exit" ("Enum"), error in (no error)=w178) -> (queue out=w180:refnum<queue>, error out=w177:errorcluster)  [unwired: 1 in, 1 out]
      }
    }
  }
  n51 = while {
    tunnel: w48 -> [w191]
    tunnel: w47 -> [w188]
    stop <- w185 stop-if-true
    # "Status Loop for Action Queues"
    n52 = Get Queue Status(queue=w191, return elements? (F)=TRUE) -> (error out=w187:errorcluster, # elements in queue=→"Action Queue Items":i32, elements=→"Action Queues items":string[])  [unwired: 1 in, 5 out]
    n53 = Get Queue Status(queue=w188, return elements? (F)=TRUE) -> (# pending remove=→"State Logic Queue Items":i32, error out=w186:errorcluster, elements=→"elements":T7[])  [unwired: 1 in, 5 out]
    n54 = Merge Errors(w187, w186) -> (w185:errorcluster)
    n55 = Wait (ms)(milliseconds to wait=u32 500) -> ()  [unwired: 1 out]
  }
  n56 = call "IMAQ Create"("Image Name"="Image dest") -> ("New Image"=w19:T22, "error out"=w18:errorcluster)  [unwired: 4 in]
  n57 = while {
    tunnel: w47 -> [w225]
    tunnel: w48 -> [w237]
    tunnel: w51 -> [w235]
    tunnel: [w234] -> _
    tunnel: [w233] -> w41
    shift-right: [w226] -> _
    shift-left: T14 {"PING_A"=0, "PING_B"=0, "PING_C"=0, "PING_D"=0} -> [w228]
    shift-right: [w219] -> _
    shift-left: State_Type_Definitions."Startup" ("Enum") -> [w222]
    shift-right: [w215] -> _
    shift-left: T15 {"xDistance"=0.0, "yDistance"=0.0, "wDistance"=0.0} -> [w217]
    shift-right: [w212] -> _
    shift-left: _ -> [w211]
    tunnel: w19 -> [w210]
    tunnel: w18 -> [w209]
    shift-right: [w206] -> _
    shift-left: T13 {"Recognized Object"=FALSE, "Object X coordinate"=0.0, "Object Y coordinate"=0.0} -> [w208]
    shift-right: [w203] -> _
    shift-left: T11 {"y Stepper Position"=0, "z Stepper Position"=0} -> [w205]
    shift-right: [w200] -> _
    shift-left: T10 {"Yaw"=0.0, "Compass"=0.0} -> [w202]
    shift-right: [w197] -> _
    shift-left: T9 {"Time up flag"=FALSE, "SET TIME TO CHECK"=0.0} -> [w199]
    shift-right: [w195] -> _
    shift-left: T8 {"yStepper desired"=0} -> [w196]
    stop <- w224 stop-if-true
    # ">>> yStepper command>>>"
    # ">>True Stop Next State >>"
    # ">>Error  >>"
    # ">>Timeout>>"
    # ">>Action states Queue Reference >>"
    # ">>State Logic Queue Reference >>"
    # "TOP LEVEL BASELINE (MAIN PROCESSING LOOP)"
    n58 = Dequeue Element(queue=w237, timeout in ms (-1)=0, error in (no error)=w235) -> (queue out=w229:refnum<queue>, element=w236:string, error out=w230:errorcluster)  [unwired: 1 out]
    "Action State" <- w236
    n59 = Wait (ms)(milliseconds to wait=u32 10) -> ()  [unwired: 1 out]
    n60 = case shown="\"REVERSE\"" w236 {
      tunnel: [_ _ _ _ _ _ _ _ _ _ _ _ _ _ _ _ 0 w1145 _ _ _ _ _ _ _ _ _ _ _ _ _ _ _ _ _ _ _ _ _ _] -> w232
      tunnel: w229 -> [_ _ _ _ _ _ _ _ _ _ _ _ _ _ _ _ _ _ _ _ _ _ _ _ _ _ _ _ _ _ _ _ _ _ _ _ _ _ _ _]
      tunnel: w228 -> [w960 w968 w979 w990 w1000 w1010 w1021 w1032 w1042 w1048 w1062 w1075 w1086 w1094 w1118 w1127 w1137 w1146 w1154 w1163 w1192 w1202 w1209 w1217 w1229 w1241 w1250 w1258 w1274 w1282 w1292 w1301 w1310 w1319 w1325 w1336 w1351 w1356 w1367 w1377]
      tunnel: [w960 w968 w979 w990 w1000 w1010 w1021 w1032 w1042 w1048 w1062 w1076 w1086 w1094 w1119 w1127 w1137 w1146 w1154 w1163 w1191 w1202 w1209 w1217 w1229 w1241 w1250 w1258 w1274 w1282 w1292 w1301 w1310 w1319 w1325 w1336 w1351 w1356 w1367 w1377] -> w227
      tunnel: [TRUE TRUE _ _ _ _ _ _ _ _ _ _ _ _ _ _ _ _ _ _ _ _ _ _ _ _ _ _ _ _ _ _ _ _ _ _ _ _ _ _] -> w224
      tunnel: w222 -> [w958 w966 w978 w989 w999 w1009 w1020 w1031 w1041 w1047 w1061 w1074 w1085 w1093 w1117 w1126 w1134 w1143 w1153 w1162 w1190 w1201 w1208 w1216 w1228 w1240 w1249 w1257 w1273 w1281 w1291 w1300 w1309 w1318 w1324 w1335 w1350 w1355 w1366 w1376]
      tunnel: [_ _ _ _ _ _ _ _ _ _ _ _ _ _ _ _ _ TRUE _ _ _ _ _ _ _ _ _ _ _ _ _ _ _ _ _ _ _ _ _ _] -> w221
      tunnel: [w958 w966 w978 w989 w999 w1009 w1020 w1031 w1041 w1047 w1061 w1074 w1085 w1093 w1117 w1126 w1134 w1143 w1153 w1162 w1190 w1201 w1208 w1216 w1228 w1240 w1249 w1257 w1273 w1281 w1291 w1300 w1309 w1318 w1324 w1335 w1350 w1355 w1366 w1376] -> w220
      tunnel: w217 -> [w957 w965 w977 w988 w998 w1008 w1019 w1030 w1040 w1049 w1060 w1073 w1087 w1095 w1116 w1128 w1133 w1142 w1155 w1164 w1180 w1200 w1211 w1218 w1230 w1242 w1251 w1259 w1275 w1284 w1294 w1303 w1312 w1321 w1327 w1338 w1353 w1358 w1369 w1379]
      tunnel: [w957 w965 w977 w988 w998 w1008 w1019 w1030 w1040 w1049 w1059 w1073 w1087 w1095 w1115 w1128 w1133 w1142 w1155 w1164 w1179 w1200 w1211 w1218 w1230 w1242 w1251 w1259 w1275 w1284 w1294 w1303 w1312 w1321 w1327 w1338 w1353 w1358 w1369 w1379] -> w216
      tunnel: w210 -> [w952 _ _ _ _ _ _ _ _ _ _ _ _ _ _ _ _ _ _ _ _ _ _ _ _ _ _ _ w1269 _ _ _ _ _ _ _ _ _ _ _]
      tunnel: w209 -> [_ _ _ _ _ _ _ _ _ _ _ _ _ _ _ _ _ _ _ _ _ _ _ _ _ _ w1243 _ w1271 w1280 _ _ _ _ _ _ _ _ _ _]
      tunnel: w208 -> [w956 w964 w976 w987 w997 w1007 w1018 w1029 w1038 w1046 w1058 w1072 w1080 w1092 w1107 w1125 w1132 w1141 w1152 w1161 w1185 w1198 w1210 w1215 w1227 w1239 w1245 w1256 w1266 w1283 w1293 w1302 w1311 w1320 w1326 w1337 w1352 w1357 w1368 w1378]
      tunnel: [w956 w964 w976 w987 w997 w1007 w1018 w1029 w1038 w1046 w1058 w1072 w1080 w1092 w1106 w1125 w1132 w1141 w1152 w1161 w1184 w1198 w1210 w1215 w1227 w1239 w1245 w1256 w1265 w1283 w1293 w1302 w1311 w1320 w1326 w1337 w1352 w1357 w1368 w1378] -> w207
      tunnel: w205 -> [w955 w963 w975 w986 w996 w1006 w1017 w1028 w1037 w1045 w1057 w1071 w1088 w1091 w1112 w1124 w1131 w1140 w1151 w1160 w1175 w1197 w1207 w1214 w1226 w1238 w1248 w1255 w1276 w1285 w1290 w1299 w1308 w1317 w1328 w1339 w1349 w1359 w1370 w1380]
      tunnel: [w955 w963 w975 w986 w996 w1006 w1017 w1028 w1037 w1045 w1057 w1071 w1088 w1091 w1111 w1124 w1131 w1140 w1151 w1160 w1174 w1197 w1207 w1214 w1226 w1238 w1248 w1255 w1276 w1285 w1290 w1299 w1308 w1317 w1328 w1339 w1348 w1359 w1370 w1380] -> w204
      tunnel: w202 -> [w954 w962 w973 w984 w994 w1005 w1015 w1026 w1036 w1044 w1056 w1064 w1083 w1090 w1102 w1123 w1130 w1139 w1150 w1159 w1171 w1196 w1204 w1213 w1225 w1237 w1247 w1254 w1277 w1286 w1289 w1296 w1305 w1314 w1329 w1340 w1343 w1360 w1371 w1381]
      tunnel: [w954 w962 w973 w984 w994 w1005 w1015 w1026 w1036 w1044 w1056 w1064 w1082 w1090 w1101 w1123 w1130 w1139 w1150 w1159 w1170 w1196 w1204 w1213 w1225 w1237 w1247 w1254 w1277 w1286 w1289 w1296 w1305 w1314 w1329 w1340 w1343 w1360 w1371 w1381] -> w201
      tunnel: w199 -> [w951 w961 w974 w985 w995 w1004 w1016 w1027 w1035 w1043 w1055 w1063 w1079 w1089 w1098 w1120 w1129 w1138 w1149 w1158 w1168 w1194 w1203 w1212 w1224 w1236 w1246 w1253 w1278 w1287 w1288 w1295 w1304 w1313 w1330 w1341 w1342 w1354 w1365 w1375]
      tunnel: [w951 w961 w974 w985 w995 w1004 w1016 w1027 w1035 w1043 w1055 w1063 w1079 w1089 w1098 w1120 w1129 w1138 w1149 w1158 w1167 w1194 w1203 w1212 w1224 w1236 w1246 w1253 w1278 w1287 w1288 w1295 w1304 w1313 w1330 w1341 w1342 w1354 w1363 w1374] -> w198
      tunnel: w196 -> [_ _ _ _ _ _ _ _ _ _ _ _ _ _ _ _ _ _ _ _ _ _ _ _ _ _ _ _ _ _ _ _ _ _ _ w1332 _ _ _ _]
      frame "Exit" {
        # ">>State Logic  >>"
        # ">>> Time cluster >>>"
        # ">>> Yaw >>>"
        # ">>> Stepper position >>>"
        # ">>> Encoders >>>"
        # ">>> Object detection >>>"
        # ">>> Ultrasonic Sensors Detect >>>"
        n61 = call "Imaq Dispose"("All Images? (No)"=TRUE, "Image"=w952) -> ()  [unwired: 4 in, 1 out]
      }
      frame "----Movement States----" {
        # ">>State Logic  >>"
        # ">>> Time cluster >>>"
        # ">>> Yaw >>>"
        # ">>> Stepper position >>>"
        # ">>> Encoders >>>"
        # ">>> Object detection >>>"
        # ">>> Ultrasonic Sensors Detect >>>"
      }
      frame "FORWARD" {
        # ">>> Time cluster >>>"
        # ">>> Yaw >>>"
        # ">>> Stepper position >>>"
        # ">>> Encoders >>>"
        # ">>> Object detection >>>"
        # ">>> Ultrasonic Sensors Detect >>>"
        n62 = Unbundle By Name(w973) -> ("Yaw"=w969:dbl)
        n63 = call "MOTOR CONTROL WITH PID AE.vi"("Yaw"=w969, "Speed"=50.0, "Direction"=MOTOR_CONTROL_WITH_PID_AE_DIRECTION_TYPE_DEF."y-axis movement", "AE Mode"=MOTOR_CONTROL_WITH_PID_AE_DATA_MODE_TYPE_DEF."Write to AE") -> ()  [unwired: 1 out]
      }
      frame "LEFT" {
        # ">>State Logic  >>"
        # ">>> Time cluster >>>"
        # ">>> Yaw >>>"
        # ">>> Stepper position >>>"
        # ">>> Encoders >>>"
        # ">>> Object detection >>>"
        # ">>> Ultrasonic Sensors Detect >>>"
        n64 = Unbundle By Name(w984) -> ("Yaw"=w981:dbl)
        n65 = call "MOTOR CONTROL WITH PID AE.vi"("Yaw"=w981, "Speed"=-25.0, "Direction"=MOTOR_CONTROL_WITH_PID_AE_DIRECTION_TYPE_DEF."x-axis movement", "AE Mode"=MOTOR_CONTROL_WITH_PID_AE_DATA_MODE_TYPE_DEF."Write to AE") -> ()  [unwired: 1 out]
      }
      frame "R-ACW" {
        # ">>> Time cluster >>>"
        # ">>> Yaw >>>"
        # ">>> Stepper position >>>"
        # ">>> Encoders >>>"
        # ">>> Object detection >>>"
        # ">>> Ultrasonic Sensors Detect >>>"
        n66 = call "MOTOR CONTROL WITH PID AE.vi"("Speed"=150.0, "Direction"=MOTOR_CONTROL_WITH_PID_AE_DIRECTION_TYPE_DEF."rotation", "AE Mode"=MOTOR_CONTROL_WITH_PID_AE_DATA_MODE_TYPE_DEF."Write to AE") -> ()  [unwired: 1 in, 1 out]
      }
      frame "R-CW" {
        (unwired) -0.2 ("Speed")
        # ">>> Time cluster >>>"
        # ">>> Yaw >>>"
        # ">>> Stepper position >>>"
        # ">>> Encoders >>>"
        # ">>> Object detection >>>"
        # ">>> Ultrasonic Sensors Detect >>>"
        n67 = call "MOTOR CONTROL WITH PID AE.vi"("Speed"=80.0, "Direction"=MOTOR_CONTROL_WITH_PID_AE_DIRECTION_TYPE_DEF."rotation", "AE Mode"=MOTOR_CONTROL_WITH_PID_AE_DATA_MODE_TYPE_DEF."Write to AE") -> ()  [unwired: 1 in, 1 out]
      }
      frame "RIGHT" {
        # ">>> Time cluster >>>"
        # ">>> Yaw >>>"
        # ">>> Stepper position >>>"
        # ">>> Encoders >>>"
        # ">>> Object detection >>>"
        # ">>> Ultrasonic Sensors Detect >>>"
        n68 = Unbundle By Name(w1015) -> ("Yaw"=w1011:dbl)
        n69 = call "MOTOR CONTROL WITH PID AE.vi"("Yaw"=w1011, "Speed"=50.0, "Direction"=MOTOR_CONTROL_WITH_PID_AE_DIRECTION_TYPE_DEF."x-axis movement", "AE Mode"=MOTOR_CONTROL_WITH_PID_AE_DATA_MODE_TYPE_DEF."Write to AE") -> ()  [unwired: 1 out]
      }
      frame "REVERSE" {
        # ">>> Time cluster >>>"
        # ">>> Yaw >>>"
        # ">>> Stepper position >>>"
        # ">>> Encoders >>>"
        # ">>> Object detection >>>"
        # ">>> Ultrasonic Sensors Detect >>>"
        n70 = Unbundle By Name(w1026) -> ("Yaw"=w1022:dbl)
        n71 = call "MOTOR CONTROL WITH PID AE.vi"("Yaw"=w1022, "Speed"=-50.0, "Direction"=MOTOR_CONTROL_WITH_PID_AE_DIRECTION_TYPE_DEF."y-axis movement", "AE Mode"=MOTOR_CONTROL_WITH_PID_AE_DATA_MODE_TYPE_DEF."Write to AE") -> ()  [unwired: 1 out]
      }
      frame "STOP" {
        n72 = Wait (ms)(milliseconds to wait=u32 100) -> ()  [unwired: 1 out]
        n73 = call "MOTOR CONTROL WITH PID AE.vi"("Direction"=MOTOR_CONTROL_WITH_PID_AE_DIRECTION_TYPE_DEF."stop", "AE Mode"=MOTOR_CONTROL_WITH_PID_AE_DATA_MODE_TYPE_DEF."Write to AE") -> ()  [unwired: 2 in, 1 out]
      }
      frame "----SENSOR READING---- " {
      }
      frame "READ ENCODERS" {
        # ">>> Time cluster >>>"
        # ">>> Yaw >>>"
        # ">>> Stepper position >>>"
        # ">>> Object detection >>>"
        # ">>> Current encoder distance >>>"
        # ">>> Ultrasonic Sensors Detect >>>"
        n74 = call "MOTOR CONTROL WITH PID AE.vi"("AE Mode"=MOTOR_CONTROL_WITH_PID_AE_DATA_MODE_TYPE_DEF."Read from AE") -> ("Speed & distance"=w1053:T1)  [unwired: 3 in]
        n75 = Unbundle By Name(w1053) -> ("xDistance"=w1052:dbl, "yDistance"=w1051:dbl, "wDistance"=w1050:dbl)
        n76 = Bundle By Name(cluster=w1060, "xDistance"=w1052, "yDistance"=w1051, "wDistance"=w1050) -> (w1059:T15)
      }
      frame "READ ULTRASONIC" {
        (unwired) navX_type_def."Read Values" ("Mode")
        (unwired) MOTOR_CONTROL_NO_PID_Type_Def."Latch" ("Direction")
        # ">>> Ultrasonic Sensors Detect >>>"
        # ">>> Object detection >>>"
        # ">>> Encoders >>>"
        # ">>> Stepper position >>>"
        # ">>> Yaw >>>"
        n77 = call "Arduino Interfacing VI.vi"("AE Mode"=Arduino_Interfacing."Read From Arduino") -> ("Arduino Data"=w1069:T4)  [unwired: 3 in, 1 out]
        n78 = Unbundle By Name(w1069) -> ("PING A"=w1068:u8, "PING B"=w1067:u8, "PING C"=w1066:u8, "PING D"=w1065:u8)
        n79 = Bundle By Name(cluster=w1075, "PING_A"=w1068, "PING_B"=w1067, "PING_C"=w1066, "PING_D"=w1065) -> (w1076:T14)
      }
      frame "READ YAW" {
        # ">>> Time cluster >>>"
        # ">>> Yaw >>>"
        # ">>> Ultrasonic Sensors Detect >>>"
        # ">>> Object detection >>>"
        # ">>> Encoders >>>"
        # ">>> Stepper position >>>"
        n80 = call "navX reading VI.vi"("Mode"=navX_type_def."Read Values") -> ("NavX Readings"=w1078:T3)  [unwired: 2 in, 3 out]
        n81 = Unbundle By Name(w1078) -> ("Heading"=w1077:dbl)
        n82 = Unbundle By Name(w1078) -> ("Yaw"=w1081:dbl)
        n83 = Bundle By Name(cluster=w1083, "Yaw"=w1081, "Compass"=w1077) -> (w1082:T10)
      }
      frame "----SYSTEM MODES----" {
        (unwired) I2C_MASTER_Type_Def."Last State" ("Arduino Mode")
        # ">>> Object detection >>>"
        # ">>> Yaw >>>"
        # ">>> Ultrasonic Sensors Detect >>>"
        # ">>> Encoders >>>"
        # ">>> Stepper position >>>"
      }
      frame "INIT" {
        w1113 = u8 0
        w1114 = 0.0
        # ">>> Time cluster >>>"
        # ">>> Object detection >>>"
        # ">>> Yaw >>>"
        # ">>> Ultrasonic Sensors Detect >>>"
        # ">>> Encoders >>>"
        # ">>> Stepper position >>>"
        # ">>State Logic  >>"
        n84 = call "Arduino Interfacing VI.vi"("AE Mode"=Arduino_Interfacing."Initialize") -> ()  [unwired: 3 in, 2 out]
        n85 = call "FGV Bool.vi"("Init/Read/Write State"=States_for_Action_Engine."Initialize") -> ()  [unwired: 2 in, 2 out]
        n86 = call "Elasped Timer.vi"("Action"=Elapsed_timer_control."Initialize") -> ()  [unwired: 7 in, 4 out]
        n87 = call "MOTOR CONTROL WITH PID AE.vi"("AE Mode"=MOTOR_CONTROL_WITH_PID_AE_DATA_MODE_TYPE_DEF."Init AE") -> ()  [unwired: 3 in, 1 out]
        n88 = Bundle By Name(cluster=w1107, "Recognized Object"=FALSE, "Object X coordinate"=0.0, "Object Y coordinate"=0.0) -> (w1106:T13)
        n89 = Bundle By Name(cluster=w1112, "y Stepper Position"=u8 0, "z Stepper Position"=u8 0) -> (w1111:T11)
        n90 = Bundle By Name(cluster=w1116, "xDistance"=w1114, "yDistance"=w1114, "wDistance"=w1114) -> (w1115:T15)
        n91 = Bundle By Name(cluster=w1118, "PING_A"=w1113, "PING_B"=w1113, "PING_C"=w1113, "PING_D"=w1113) -> (w1119:T14)
        n92 = Bundle By Name(cluster=w1102, "Yaw"=0.0) -> (w1101:T10)
      }
      frame "ARDUINO - ULTRASONIC" {
        # ">>> Object detection >>>"
        # ">>> Yaw >>>"
        # ">>> Ultrasonic Sensors Detect >>>"
        # ">>> Encoders >>>"
        # ">>> Stepper position >>>"
        # ">>State Logic  >>"
        n93 = call "Arduino Interfacing VI.vi"("Data to Write"=I2C_MASTER_WRITE_NEW_Type_Def."Ultrasonic sensors", "AE Mode"=Arduino_Interfacing."Write to Arduino") -> ()  [unwired: 2 in, 2 out]
      }
      frame "NAVX CALIBRATE" {
        # ">>> Object detection >>>"
        # ">>> Yaw >>>"
        # ">>> Ultrasonic Sensors Detect >>>"
        # ">>> Encoders >>>"
        # ">>> Stepper position >>>"
        # ">>State Logic  >>"
        # "Adds a 15 second delay to the startup process \nfor the NavX to calibrate"
        n94 = Wait (ms)(milliseconds to wait=u32 5000) -> ()  [unwired: 1 out]
      }
      frame "NO ACTION", Default {
        (unwired) u8 0 ("y Stepper value")
        (unwired) TRUE ("Latch")
        (unwired) navX_type_def."Read Values" ("Mode")
        (unwired) MOTOR_CONTROL_NO_PID_Type_Def."Latch" ("Direction")
        # ">>> Object detection >>>"
        # ">>> Yaw >>>"
        # ">>> Ultrasonic Sensors Detect >>>"
        # ">>> Encoders >>>"
        # ">>> Stepper position >>>"
        # ">>State Logic  >>"
        n95 = case shown="4" w1143 {
          tunnel: [0 100] -> w1145
          frame 1, Default {
          }
          frame 4 {
          }
        }
      }
      frame "----RESET CASES----" {
        (unwired) I2C_MASTER_Type_Def."Last State" ("Arduino Mode")
        # ">>> Object detection >>>"
        # ">>> Yaw >>>"
        # ">>> Ultrasonic Sensors Detect >>>"
        # ">>> Encoders >>>"
        # ">>> Stepper position >>>"
        # ">>State Logic  >>"
      }
      frame "RESET ENCODERS" {
        # ">>> Object detection >>>"
        # ">>> Yaw >>>"
        # ">>> Ultrasonic Sensors Detect >>>"
        # ">>> Encoders >>>"
        # ">>> Stepper position >>>"
        # ">>State Logic  >>"
        n96 = call "MOTOR CONTROL WITH PID AE.vi"("Direction"=MOTOR_CONTROL_WITH_PID_AE_DIRECTION_TYPE_DEF."reset encoders", "AE Mode"=MOTOR_CONTROL_WITH_PID_AE_DATA_MODE_TYPE_DEF."Write to AE") -> ()  [unwired: 2 in, 1 out]
      }
      frame "RESET FLAGS" {
        (unwired) I2C_MASTER_Type_Def."Last State" ("Arduino Mode")
        # "Resets any software variables\nand/or non-critical states"
        n97 = Wait (ms)(milliseconds to wait=u32 20) -> ()  [unwired: 1 out]
        n98 = Bundle By Name(cluster=w1168, "Time up flag"=FALSE, "SET TIME TO CHECK"=0.0) -> (w1167:T9)
        n99 = Bundle By Name(cluster=w1185, "Recognized Object"=FALSE, "Object X coordinate"=0.0, "Object Y coordinate"=0.0) -> (w1184:T13)
        n100 = Bundle By Name(cluster=w1175, "y Stepper Position"=u8 0, "z Stepper Position"=u8 0) -> (w1174:T11)
        n101 = Bundle By Name(cluster=w1180, "xDistance"=0.0, "yDistance"=0.0, "wDistance"=0.0) -> (w1179:T15)
        n102 = Bundle By Name(cluster=w1192, "PING_A"=u8 0, "PING_B"=u8 0, "PING_C"=u8 0, "PING_D"=u8 0) -> (w1191:T14)
        n103 = Bundle By Name(cluster=w1171, "Yaw"=0.0) -> (w1170:T10)
      }
      frame "RESET YAW" {
        n104 = Wait (ms)(milliseconds to wait=u32 100) -> ()  [unwired: 1 out]
        n105 = call "navX reading VI.vi"("Mode"=navX_type_def."Zero Yaw") -> ()  [unwired: 2 in, 4 out]
      }
      frame "RESET ARM" {
        n106 = call "Arduino Interfacing VI.vi"("Data to Write"=I2C_MASTER_WRITE_NEW_Type_Def."Soft Reset", "AE Mode"=Arduino_Interfacing."Write to Arduino") -> ()  [unwired: 2 in, 2 out]
      }
      frame "--------CAM STATES-------" {
      }
      frame "OPEN LOG CAM" {
        n107 = call "Webcam AE.vi"("Session In"=T29 "cam0", "Camera states"=Webcam_AE."Initialize Camera") -> ("error out"=w1221:errorcluster, "Session Out"=w1220:T29)  [unwired: 1 in, 1 out]
        n108 = call "Webcam AE.vi"("error in (no error)"=w1221, "Session In"=w1220, "Camera states"=Webcam_AE."Open Camera") -> ()  [unwired: 3 out]
      }
      frame "OPEN LIFE CAM" {
        n109 = call "Webcam AE.vi"("Session In"=T29 "cam1", "Camera states"=Webcam_AE."Initialize Camera") -> ("error out"=w1233:errorcluster, "Session Out"=w1232:T29)  [unwired: 1 in, 1 out]
        n110 = call "Webcam AE.vi"("error in (no error)"=w1233, "Session In"=w1232, "Camera states"=Webcam_AE."Open Camera") -> ()  [unwired: 3 out]
      }
      frame "CAM ACQ" {
        # ">>State Logic  >>"
        # ">>> Time cluster >>>"
        # ">>> Yaw >>>"
        # ">>> Stepper position >>>"
        # ">>> Encoders >>>"
        # ">>> Object detection >>>"
        # ">>> Ultrasonic Sensors Detect >>>"
        n111 = call "Webcam AE.vi"("error in (no error)"=w1243, "Camera states"=Webcam_AE."Continuous Acquisition") -> ()  [unwired: 1 in, 3 out]
      }
      frame "CAM CLOSE" {
        # ">>State Logic  >>"
        # ">>> Time cluster >>>"
        # ">>> Yaw >>>"
        # ">>> Stepper position >>>"
        # ">>> Encoders >>>"
        # ">>> Object detection >>>"
        # ">>> Ultrasonic Sensors Detect >>>"
        n112 = call "Webcam AE.vi"("Camera states"=Webcam_AE."Close Camera") -> ()  [unwired: 2 in, 3 out]
      }
      frame "PROCESS IMAGE" {
        # ">>State Logic  >>"
        # ">>> Time cluster >>>"
        # ">>> Yaw >>>"
        # ">>> Stepper position >>>"
        # ">>> Encoders >>>"
        # ">>> Object detection >>>"
        # ">>> Ultrasonic Sensors Detect >>>"
        n113 = call "Webcam AE.vi"("error in (no error)"=w1271, "Camera states"=Webcam_AE."Retrieve Image") -> ("error out"=w1267:errorcluster, "Image Out"=w1270:T22)  [unwired: 1 in, 1 out]
        n114 = call "Object Detection SubVI.vi"("Error In"=w1267, "Mode"="Object recognition mode", "Image Dest"=w1269, "Image in"=w1270) -> ("Object Center Coordinates"=w1264:cluster{"x":sgl, "y":sgl}, "Object detection cluster"=w1260:T2)  [unwired: 2 out]
        "Object detection cluster" <- w1260
        "Object Center Coordinates" <- w1264
        n115 = Unbundle By Name(w1260) -> ("Object detected?"=w1261:bool)
        n116 = Unbundle By Name(w1264) -> ("x"=w1263:sgl, "y"=w1262:sgl)
        n117 = Bundle By Name(cluster=w1266, "Recognized Object"=w1261, "Object X coordinate"=w1263, "Object Y coordinate"=w1262) -> (w1265:T13)
      }
      frame "DISPOSE BUFFERS" {
        # ">>State Logic  >>"
        # ">>> Time cluster >>>"
        # ">>> Yaw >>>"
        # ">>> Stepper position >>>"
        # ">>> Encoders >>>"
        # ">>> Object detection >>>"
        # ">>> Ultrasonic Sensors Detect >>>"
        n118 = call "Webcam AE.vi"("error in (no error)"=w1280, "Camera states"=Webcam_AE."Dispose Image Buffers") -> ()  [unwired: 1 in, 3 out]
      }
      frame "-----ARM ACTIONS-----" {
      }
      frame "CLOSE CLAW" {
        n119 = call "Arduino Interfacing VI.vi"("Data to Write"=I2C_MASTER_WRITE_NEW_Type_Def."Close Claw", "AE Mode"=Arduino_Interfacing."Write to Arduino") -> ()  [unwired: 2 in, 2 out]
      }
      frame "OPEN CLAW" {
        n120 = call "Arduino Interfacing VI.vi"("Data to Write"=I2C_MASTER_WRITE_NEW_Type_Def."Open Claw", "AE Mode"=Arduino_Interfacing."Write to Arduino") -> ()  [unwired: 2 in, 2 out]
      }
      frame "Z STEPPER CAM HEIGHT" {
        n121 = call "Arduino Interfacing VI.vi"("Data to Write"=I2C_MASTER_WRITE_NEW_Type_Def."zStepper 8k", "AE Mode"=Arduino_Interfacing."Write to Arduino") -> ()  [unwired: 2 in, 2 out]
      }
      frame "Z STEPPER GRAB HEIGHT" {
        # ">>State Logic  >>"
        # ">>> Time cluster >>>"
        # ">>> Yaw >>>"
        # ">>> Stepper position >>>"
        # ">>> Encoders >>>"
        # ">>> Object detection >>>"
        # ">>> Ultrasonic Sensors Detect >>>"
        n122 = call "Arduino Interfacing VI.vi"("Data to Write"=I2C_MASTER_WRITE_NEW_Type_Def."zStepper 100", "AE Mode"=Arduino_Interfacing."Write to Arduino") -> ()  [unwired: 2 in, 2 out]
      }
      frame "Y STEPPER CONTROL" {
        # ">>State Logic  >>"
        # ">>> yStepper command>>>"
        # ">>> Time cluster >>>"
        # ">>> Yaw >>>"
        # ">>> Stepper position >>>"
        # ">>> Encoders >>>"
        # ">>> Object detection >>>"
        # ">>> Ultrasonic Sensors Detect >>>"
        n123 = Unbundle By Name(w1332) -> ("yStepper desired"=w1331:u8)
        n124 = call "Arduino Interfacing VI.vi"("y Stepper value"=w1331, "Data to Write"=I2C_MASTER_WRITE_NEW_Type_Def."yStepper control", "AE Mode"=Arduino_Interfacing."Write to Arduino") -> ()  [unwired: 1 in, 2 out]
      }
      frame "READ STEPPER VALUES" {
        # ">>State Logic  >>"
        # ">>> Time cluster >>>"
        # ">>> Yaw >>>"
        # ">>> Stepper position >>>"
        # ">>> Encoders >>>"
        # ">>> Object detection >>>"
        # ">>> Ultrasonic Sensors Detect >>>"
        n125 = call "Arduino Interfacing VI.vi"("AE Mode"=Arduino_Interfacing."Read From Arduino") -> ("Arduino Data"=w1346:T4)  [unwired: 3 in, 1 out]
        n126 = Unbundle By Name(w1346) -> ("y Stepper Position"=w1345:u8, "z Stepper Position"=w1344:u8)
        n127 = Bundle By Name(cluster=w1349, "y Stepper Position"=w1345, "z Stepper Position"=w1344) -> (w1348:T11)
      }
      frame " -----TIMING-----" {
        # ">>State Logic  >>"
        # ">>> Time cluster >>>"
        # ">>> Yaw >>>"
        # ">>> Stepper position >>>"
        # ">>> Encoders >>>"
        # ">>> Object detection >>>"
        # ">>> Ultrasonic Sensors Detect >>>"
      }
      frame "SET TIMER" {
        # ">>State Logic  >>"
        # ">>> Time cluster >>>"
        # ">>> Yaw >>>"
        # ">>> Stepper position >>>"
        # ">>> Encoders >>>"
        # ">>> Object detection >>>"
        # ">>> Ultrasonic Sensors Detect >>>"
        n128 = call "Elasped Timer.vi"("Time Setting"=5.0, "Action"=Elapsed_timer_control."Initialize") -> ()  [unwired: 6 in, 4 out]
        n129 = Bundle By Name(cluster=w1365, "Time up flag"=FALSE) -> (w1363:T9)
      }
      frame "START TIMER" {
        # ">>State Logic  >>"
        # ">>> Time cluster >>>"
        # ">>> Yaw >>>"
        # ">>> Stepper position >>>"
        # ">>> Encoders >>>"
        # ">>> Object detection >>>"
        # ">>> Ultrasonic Sensors Detect >>>"
        n130 = call "Elasped Timer.vi"("Action"=Elapsed_timer_control."Start") -> ("Time Out?!"=w1372:bool)  [unwired: 7 in, 3 out]
        n131 = Bundle By Name(cluster=w1375, "Time up flag"=w1372) -> (w1374:T9)
      }
    }
    "State Logic" <- w220
    n132 = local read "TASK ENABLE"() -> (w214:bool)
    n133 = Not(x=w214) -> (.not. x?=w213:bool)
    n134 = case shown="True" w221 {
      tunnel: w225 -> [w248 w279]
      tunnel: w229 -> [w244 w281]
      tunnel: [w248 w279] -> w234
      tunnel: [w244 w282] -> w233
      tunnel: w230 -> [_ w277]
      tunnel: w232 -> [_ w278]
      tunnel: w227 -> [w247 w284]
      tunnel: [w247 w284] -> w226
      tunnel: "STOP TASK" -> [_ w267]
      tunnel: w220 -> [w246 w283]
      tunnel: [w246 w280] -> w219
      tunnel: w216 -> [w245 w273]
      tunnel: [w245 w273] -> w215
      tunnel: w213 -> [_ w268]
      tunnel: [w243 w265] -> w212
      tunnel: w211 -> [w243 w264]
      tunnel: w207 -> [w242 w261]
      tunnel: [w242 w261] -> w206
      tunnel: w204 -> [w241 w257]
      tunnel: [w241 w257] -> w203
      tunnel: w201 -> [w240 w255]
      tunnel: [w240 w255] -> w200
      tunnel: w198 -> [w239 w253]
      tunnel: [w239 w253] -> w197
      tunnel: w196 -> [w238 w252]
      tunnel: [w238 w251] -> w195
      tunnel: [_ w249] -> w194
      frame False {
        # ">>> yStepper command>>>"
        # ">>> Time cluster >>>"
        # ">>> Yaw >>>"
        # ">>> Stepper position >>>"
        # ">>> Encoders >>>"
        # ">>> Object detection >>>"
        # ">>> Ultrasonic Sensors Detect >>>"
        # ">>> Time cluster >>>"
        # ">>> Yaw >>>"
        # ">>> Stepper position >>>"
        # ">>> Encoders >>>"
        # ">>> Object detection >>>"
        # ">>> Ultrasonic Sensors Detect >>>"
      }
      frame True {
        # ">>State Logic Queue Reference >>"
        # ">>Timeout>>"
        # ">>> yStepper command>>>"
        # ">>> Time cluster >>>"
        # ">>> Object detection >>>"
        # ">>> Yaw >>>"
        # ">>> Ultrasonic Sensors Detect >>>"
        # ">>> Encoders >>>"
        # ">>> Stepper position >>>"
        # ">>State Logic  >>"
        # ">>True Stop Next State >>"
        # ">>Action Queue>>"
        # ">> Manual override >>"
        # ">>> Time cluster >>>"
        # ">>> Yaw >>>"
        # ">>> Stepper position >>>"
        # ">>> Encoders >>>"
        # ">>> Object detection >>>"
        # ">>> Ultrasonic Sensors Detect >>>"
        # ">>Action Queue>>"
        # ">>State Logic Queue Reference >>"
        n135 = Or(x=w267, y=w268) -> (x .or. y?=w266:bool)
        n136 = Unbundle By Name(w255) -> ("Yaw"=w256:dbl, "Compass"=w250:dbl)
        n137 = Unbundle By Name(w253) -> ("Time up flag"=w254:bool)
        "Time up flag" <- w254
        n138 = Unbundle By Name(w257) -> ("y Stepper Position"=w259:u8, "z Stepper Position"=w258:u8)
        n139 = Unbundle By Name(w273) -> ("xDistance"=w270:dbl, "yDistance"=w271:dbl, "wDistance"=w272:dbl)
        n140 = Unbundle By Name(w261) -> ("Recognized Object"=w260:bool, "Object X coordinate"=w263:dbl, "Object Y coordinate"=w262:dbl)
        n141 = Unbundle By Name(w284) -> ("PING_A"=w276:u8, "PING_B"=w275:u8, "PING_C"=w274:u8, "PING_D"=w269:u8)
        n142 = case shown="14" w283 {
          tunnel: [w287 w293 w305 w314 w374 w387 w424 w471 w513 w565 w611 w650 w709 w753 w792 w837 _ w881 w919] -> w282
          tunnel: w281 -> [w287 w296 w306 w317 w376 w388 w425 w472 w519 w558 w614 w657 w699 w756 w798 w836 _ w872 w914]
          tunnel: [State_Type_Definitions."Idle" ("Enum") State_Type_Definitions."Idle" ("Enum") w301 w316 State_Type_Definitions."Shutdown" ("Enum") w389 w427 w470 w514 w564 w612 w652 w708 w754 w799 w838 _ w873 w920] -> w280
          tunnel: w279 -> [_ _ w304 w320 _ w394 w437 w479 w518 w562 w615 w656 w706 w751 w797 w834 _ w880 w917]
          tunnel: w278 -> [_ _ _ w319 _ w393 w436 w478 w517 w561 w608 w655 w705 w750 w796 w833 _ w878 w916]
          tunnel: w277 -> [_ _ w303 w315 _ w392 w435 w477 w516 w560 w607 w654 w707 w752 w795 w832 _ w879 w915]
          tunnel: w266 -> [_ _ _ _ _ w386 w426 w474 w512 w563 w613 w658 w700 w757 w793 w835 _ w876 w918]
          tunnel: w276 -> [_ _ _ _ _ _ _ _ _ _ _ _ _ _ _ _ _ _ _]
          tunnel: w275 -> [_ _ _ _ _ _ w433 _ _ w554 w596 w648 _ w743 _ _ _ _ _]
          tunnel: w274 -> [_ _ _ _ _ _ w432 _ _ w555 w597 w649 _ w744 _ _ _ _ _]
          tunnel: w272 -> [_ _ _ _ _ _ _ w476 _ _ _ _ _ _ _ _ _ _ _]
          tunnel: w271 -> [_ _ _ _ _ w385 _ _ _ _ _ w653 _ _ _ _ _ _ _]
          tunnel: w270 -> [_ _ _ _ _ _ _ _ _ _ w602 _ _ _ _ _ _ _ _]
          tunnel: w269 -> [_ _ _ _ _ _ _ _ _ _ _ _ _ _ _ _ _ _ _]
          tunnel: [State_Type_Definitions."Idle" ("Enum") State_Type_Definitions."Idle" ("Enum") State_Type_Definitions."Idle" ("Enum") State_Type_Definitions."Idle" ("Enum") State_Type_Definitions."Shutdown" ("Enum") w382 w423 w467 w511 w557 w610 w651 w710 w755 w791 w839 _ w874 w921] -> w265
          tunnel: w264 -> [_ _ w301 _ _ _ _ _ _ _ _ _ _ _ _ _ _ _ _]
          tunnel: w260 -> [_ _ _ _ _ _ _ _ _ _ _ _ _ _ _ w829 _ w875 _]
          tunnel: w263 -> [_ _ _ _ _ _ _ _ _ _ _ _ _ _ _ _ _ _ _]
          tunnel: w262 -> [_ _ _ _ _ _ _ _ _ _ _ _ _ _ _ _ _ _ _]
          tunnel: w259 -> [_ _ _ _ _ _ _ _ _ _ _ _ _ _ _ _ _ _ _]
          tunnel: w258 -> [_ _ _ _ _ _ _ _ w509 _ _ _ w703 _ _ _ _ _ w913]
          tunnel: w256 -> [_ _ _ _ _ _ _ _ _ _ _ _ _ _ _ _ _ _ _]
          tunnel: w254 -> [_ _ _ _ _ _ _ _ _ _ _ _ _ _ w789 _ _ _ _]
          tunnel: w252 -> [w285 w291 w300 w312 w372 w381 w422 w466 w510 w556 w606 w647 w698 w748 w790 w830 _ w871 w910]
          tunnel: [w285 w290 w300 w312 w372 w381 w422 w466 w510 w556 w606 w647 w698 w748 w790 w830 _ w871 w910] -> w251
          tunnel: w250 -> [_ _ _ _ _ _ _ _ _ _ _ _ _ _ _ _ _ _ _]
          tunnel: [_ _ _ TRUE _ _ _ _ _ _ _ _ _ _ _ _ _ _ _] -> w249
          frame 0 {
            # ">>> yStepper command>>>"
          }
          frame 1 {
            # ">>> yStepper command>>>"
            n143 = for {
              shift-right: [w299] -> w293
              shift-left: w296 -> [w298]
              tunnel: string[] ["INIT", "RESET ARM", "RESET FLAGS", "RESET YAW", "NAVX CALIBRATE"] -> [w297] mode=indexing
              n144 = Enqueue Element(queue=w298, element=w297) -> (queue out=w299:refnum<queue>)  [unwired: 2 in, 2 out]
            }
            n145 = Bundle By Name(cluster=w291, "yStepper desired"=u8 0) -> (w290:T8)
          }
          frame 3 {
            # ">>> yStepper command>>>"
            n146 = Flush Queue(queue=w304, error in (no error)=w303) -> ()  [unwired: 3 out]
            n147 = for {
              shift-right: [w310] -> w305
              shift-left: w306 -> [w309]
              tunnel: string[] ["STOP", "RESET ENCODERS", "RESET YAW", "RESET ARM", "RESET FLAGS", "DISPOSE BUFFERS", "CAM CLOSE"] -> [w308] mode=indexing
              n148 = Enqueue Element(queue=w309, element=w308) -> (queue out=w310:refnum<queue>)  [unwired: 2 in, 2 out]
            }
          }
          frame 4, Default {
            (unwired) TRUE ("Green LED")
            # ">>> yStepper command>>>"
            n149 = Dequeue Element(queue=w320, timeout in ms (-1)=w319, error in (no error)=w315) -> (element=w318:T7)  [unwired: 3 out]
            n150 = case shown="\"Start Task 4\"" w318 {
              tunnel: [w322 w329 w336 w343 w350 w357 w364 w366] -> w314
              tunnel: w317 -> [w323 w330 w337 w344 w351 w358 w364 w367]
              tunnel: [State_Type_Definitions."Task 1" ("Enum") State_Type_Definitions."Task 2" ("Enum") State_Type_Definitions."Task 3" ("Enum") State_Type_Definitions."Task 4_A" ("Enum") State_Type_Definitions."Task 5_A" ("Enum") State_Type_Definitions."Task 6_A" ("Enum") State_Type_Definitions."Idle" ("Enum") State_Type_Definitions."Shutdown" ("Enum")] -> w316
              frame "Start Task 1" {
                n151 = for {
                  shift-right: [w327] -> w322
                  shift-left: w323 -> [w326]
                  tunnel: string[] ["RESET ENCODERS", "RESET YAW", "FORWARD", "READ ENCODERS"] -> [w325] mode=indexing
                  n152 = Enqueue Element(queue=w326, element=w325) -> (queue out=w327:refnum<queue>)  [unwired: 2 in, 2 out]
                }
              }
              frame "Start Task 2" {
                n153 = for {
                  shift-right: [w334] -> w329
                  shift-left: w330 -> [w333]
                  tunnel: string[] ["RESET ENCODERS", "RESET YAW", "READ ULTRASONIC", "ARDUINO - ULTRASONIC"] -> [w332] mode=indexing
                  n154 = Enqueue Element(queue=w333, element=w332) -> (queue out=w334:refnum<queue>)  [unwired: 2 in, 2 out]
                }
              }
              frame "Start Task 3" {
                n155 = for {
                  shift-right: [w341] -> w336
                  shift-left: w337 -> [w340]
                  tunnel: string[] ["RESET ENCODERS", "READ ENCODERS", "R-ACW"] -> [w339] mode=indexing
                  n156 = Enqueue Element(queue=w340, element=w339) -> (queue out=w341:refnum<queue>)  [unwired: 2 in, 2 out]
                }
              }
              frame "Start Task 4" {
                n157 = for {
                  shift-right: [w348] -> w343
                  shift-left: w344 -> [w347]
                  tunnel: string[] ["RESET YAW", "RESET ENCODERS", "RESET ARM", "RESET FLAGS", "", ""] -> [w346] mode=indexing
                  n158 = Enqueue Element(queue=w347, element=w346) -> (queue out=w348:refnum<queue>)  [unwired: 2 in, 2 out]
                }
              }
              frame "Start Task 5" {
                n159 = for {
                  shift-right: [w355] -> w350
                  shift-left: w351 -> [w354]
                  tunnel: string[] ["RESET YAW", "RESET ENCODERS", "READ STEPPER VALUES", "Z STEPPER CAM HEIGHT", "", ""] -> [w353] mode=indexing
                  n160 = Enqueue Element(queue=w354, element=w353) -> (queue out=w355:refnum<queue>)  [unwired: 2 in, 2 out]
                }
              }
              frame "Start Task 6" {
                n161 = for {
                  shift-right: [w362] -> w357
                  shift-left: w358 -> [w361]
                  tunnel: string[] ["OPEN LOG CAM ", "", "", "", "", ""] -> [w360] mode=indexing
                  n162 = Enqueue Element(queue=w361, element=w360) -> (queue out=w362:refnum<queue>)  [unwired: 2 in, 2 out]
                }
              }
              frame "None", Default {
              }
              frame "Exit" {
                n163 = for {
                  shift-right: [w371] -> w366
                  shift-left: w367 -> [w370]
                  tunnel: string[] ["STOP", "RESET ENCODERS", "RESET YAW", "EXIT"] -> [w369] mode=indexing
                  n164 = Enqueue Element(queue=w370, element=w369) -> (queue out=w371:refnum<queue>)  [unwired: 2 in, 2 out]
                }
              }
            }
          }
          frame 5 {
            # ">>> yStepper command>>>"
            n165 = for {
              shift-right: [w380] -> w374
              shift-left: w376 -> [w379]
              tunnel: string[] ["INIT", "RESET ENCODERS", "RESET FLAGS", "CAM CLOSE", "DISPOSE BUFFERS", "EXIT", ""] -> [w378] mode=indexing
              n166 = Enqueue Element(queue=w379, element=w378) -> (queue out=w380:refnum<queue>)  [unwired: 2 in, 2 out]
            }
          }
          frame 6 {
            # ">>> yStepper command>>>"
            # "Use 250"
            n167 = Dequeue Element(queue=w394, timeout in ms (-1)=w393, error in (no error)=w392) -> (element=w391:T7)  [unwired: 3 out]
            n168 = Greater?(x=w385, y=250.0) -> (0:w383:bool)
            n169 = Or(x=w383, y=w386) -> (x .or. y?=w390:bool)
            n170 = case shown="\"None\", Default" w391 {
              tunnel: w390 -> [w397 _]
              tunnel: [w401 State_Type_Definitions."True Stop" ("Enum")] -> w389
              tunnel: w388 -> [w398 w416]
              tunnel: [w396 w415] -> w387
              tunnel: [State_Type_Definitions."Idle" ("Enum") State_Type_Definitions."Shutdown" ("Enum")] -> w382
              frame "None", Default {
                n171 = case shown="True" w397 {
                  tunnel: w398 -> [w404 w410]
                  tunnel: [w403 w408] -> w396
                  frame False {
                    n172 = for {
                      shift-right: [w406] -> w403
                      shift-left: w404 -> [w407]
                      tunnel: string[] ["READ ENCODERS", "READ YAW", "FORWARD"] ("element") -> [w405] mode=indexing
                      n173 = Enqueue Element(queue=w407, element=w405) -> (queue out=w406:refnum<queue>)  [unwired: 2 in, 2 out]
                    }
                  }
                  frame True {
                    n174 = for {
                      shift-right: [w412] -> w408
                      shift-left: w410 -> [w413]
                      tunnel: string[] ["RESET YAW", "RESET ENCODERS", "STOP", ""] -> [w411] mode=indexing
                      n175 = Enqueue Element(queue=w413, element=w411) -> (queue out=w412:refnum<queue>)  [unwired: 2 in, 2 out]
                    }
                  }
                }
                n176 = Select(t=State_Type_Definitions."True Stop" ("Enum"), s=w397, f=State_Type_Definitions."Task 1" ("Enum")) -> (s? t:f=w401:u16)
              }
              frame "Exit" {
                n177 = for {
                  shift-right: [w420] -> w415
                  shift-left: w416 -> [w421]
                  tunnel: string[] ["STOP", "RESET ENCODERS", "RESET YAW", ""] -> [w419] mode=indexing
                  n178 = Enqueue Element(queue=w421, element=w419) -> (queue out=w420:refnum<queue>)  [unwired: 2 in, 2 out]
                }
              }
            }
          }
          frame 7 {
            w431 = u8 30 ("y")
            # ">>> yStepper command>>>"
            # ">>Object detected>>"
            n179 = Dequeue Element(queue=w437, timeout in ms (-1)=w436, error in (no error)=w435) -> (element=w434:T7)  [unwired: 3 out]
            n180 = Less?(x=w433, y=w431) -> (x < y?=w430:bool)
            n181 = Less?(x=w432, y=w431) -> (x < y?=w429:bool)
            n182 = Or(x=w430, y=w429) -> (x .or. y?=w428:bool)
            "Obstacle detected" <- w428
            n183 = case shown="\"None\", Default" w434 {
              tunnel: w428 -> [w441 _]
              tunnel: [w443 State_Type_Definitions."True Stop" ("Enum")] -> w427
              tunnel: w426 -> [w442 _]
              tunnel: w425 -> [w440 w460]
              tunnel: [w439 w461] -> w424
              tunnel: [State_Type_Definitions."Idle" ("Enum") State_Type_Definitions."Shutdown" ("Enum")] -> w423
              frame "None", Default {
                n184 = case shown="True" w441 {
                  tunnel: w440 -> [w447 w454]
                  tunnel: [w448 w453] -> w439
                  frame False {
                    n185 = for {
                      tunnel: string[] ["READ ULTRASONIC", "STOP"] ("element") -> [w449] mode=indexing
                      shift-right: [w451] -> w448
                      shift-left: w447 -> [w450]
                      n186 = Enqueue Element(queue=w450, element=w449) -> (queue out=w451:refnum<queue>)  [unwired: 2 in, 2 out]
                    }
                  }
                  frame True {
                    n187 = for {
                      shift-right: [w456] -> w453
                      shift-left: w454 -> [w457]
                      tunnel: string[] ["REVERSE", "READ ULTRASONIC", "READ YAW"] -> [w455] mode=indexing
                      n188 = Enqueue Element(queue=w457, element=w455) -> (queue out=w456:refnum<queue>)  [unwired: 2 in, 2 out]
                    }
                  }
                }
                n189 = Select(t=State_Type_Definitions."True Stop" ("Enum"), s=w442, f=State_Type_Definitions."Task 2" ("Enum")) -> (s? t:f=w443:u16)
              }
              frame "Exit" {
                n190 = for {
                  shift-right: [w464] -> w461
                  shift-left: w460 -> [w465]
                  tunnel: string[] ["STOP", "RESET ENCODERS", "RESET YAW", "ARDUINO MODE 0"] -> [w463] mode=indexing
                  n191 = Enqueue Element(queue=w465, element=w463) -> (queue out=w464:refnum<queue>)  [unwired: 2 in, 2 out]
                }
              }
            }
          }
          frame 11 {
            # ">>> yStepper command>>>"
            n192 = Dequeue Element(queue=w479, timeout in ms (-1)=w478, error in (no error)=w477) -> (element=w468:T7)  [unwired: 3 out]
            n193 = Greater?(x=w476, y=160.0) -> (0:w473:bool)
            n194 = Or(x=w473, y=w474) -> (x .or. y?=w469:bool)
            n195 = case shown="\"None\", Default" w468 {
              tunnel: w469 -> [w482 _]
              tunnel: [w486 State_Type_Definitions."True Stop" ("Enum")] -> w470
              tunnel: w472 -> [w483 w502]
              tunnel: [w481 w501] -> w471
              tunnel: [State_Type_Definitions."Idle" ("Enum") State_Type_Definitions."Shutdown" ("Enum")] -> w467
              frame "None", Default {
                n196 = case shown="False" w482 {
                  tunnel: w483 -> [w489 w495]
                  tunnel: [w488 w493] -> w481
                  frame False {
                    n197 = for {
                      shift-right: [w491] -> w488
                      shift-left: w489 -> [w492]
                      tunnel: string[] ["READ ENCODERS", "R-ACW"] ("element") -> [w490] mode=indexing
                      n198 = Enqueue Element(queue=w492, element=w490) -> (queue out=w491:refnum<queue>)  [unwired: 2 in, 2 out]
                    }
                  }
                  frame True {
                    n199 = for {
                      shift-right: [w497] -> w493
                      shift-left: w495 -> [w498]
                      tunnel: string[] ["RESET YAW", "RESET ENCODERS", "STOP", "ARDUINO MODE 0"] -> [w496] mode=indexing
                      n200 = Enqueue Element(queue=w498, element=w496) -> (queue out=w497:refnum<queue>)  [unwired: 2 in, 2 out]
                    }
                  }
                }
                n201 = Select(t=State_Type_Definitions."True Stop" ("Enum"), s=w482, f=State_Type_Definitions."Task 3" ("Enum")) -> (s? t:f=w486:T6)
              }
              frame "Exit" {
                n202 = for {
                  shift-right: [w505] -> w501
                  shift-left: w502 -> [w506]
                  tunnel: string[] ["STOP", "RESET ENCODERS", "RESET YAW", ""] -> [w504] mode=indexing
                  n203 = Enqueue Element(queue=w506, element=w504) -> (queue out=w505:refnum<queue>)  [unwired: 2 in, 2 out]
                }
              }
            }
          }
          frame 12 {
            # ">> Stepper height reeached >>"
            # ">>> yStepper command>>>"
            # ">> Manual override >>"
            n204 = Dequeue Element(queue=w518, timeout in ms (-1)=w517, error in (no error)=w516) -> (element=w515:T7)  [unwired: 3 out]
            n205 = Equal?(x=w509, y=u8 80) -> (x = y?=w507:bool)
            n206 = case shown="\"None\", Default" w515 {
              tunnel: [w530 State_Type_Definitions."True Stop" ("Enum")] -> w514
              tunnel: [w528 w545] -> w513
              tunnel: w519 -> [w527 _]
              tunnel: w512 -> [w521 _]
              tunnel: [State_Type_Definitions."Idle" ("Enum") State_Type_Definitions."Shutdown" ("Enum")] -> w511
              tunnel: w507 -> [w520 _]
              frame "None", Default {
                # ">> WIill proceed to part ii if not manual override >>"
                # ">>If ENABLE or Trigger is set to true>>"
                n207 = Or(x=w520, y=w521) -> (x .or. y?=w522:bool)
                n208 = case shown="True" w520 {
                  tunnel: [w533 w539] -> w528
                  tunnel: w527 -> [w532 w538]
                  frame False {
                    n209 = for {
                      shift-right: [w535] -> w533
                      shift-left: w532 -> [w536]
                      tunnel: string[] ["Z STEPPER CAM HEIGHT", "READ STEPPER VALUES"] ("element") -> [w534] mode=indexing
                      n210 = Enqueue Element(queue=w536, element=w534) -> (queue out=w535:refnum<queue>)  [unwired: 2 in, 2 out]
                    }
                  }
                  frame True {
                    n211 = for {
                      shift-right: [w541] -> w539
                      shift-left: w538 -> [w542]
                      tunnel: string[] ["ARDUINO - ULTRASONIC", "READ ULTRASONIC", "FORWARD", "", "", ""] -> [w540] mode=indexing
                      n212 = Enqueue Element(queue=w542, element=w540) -> (queue out=w541:refnum<queue>)  [unwired: 2 in, 2 out]
                    }
                  }
                }
                n213 = Select(t=State_Type_Definitions."True Stop" ("Enum"), s=w521, f=State_Type_Definitions."Task 4_B" ("Enum")) -> (s? t:f=w524:T6)
                n214 = Select(t=w524, s=w522, f=State_Type_Definitions."Task 4_A" ("Enum")) -> (s? t:f=w530:T6)
              }
              frame "Exit" {
                n215 = for {
                  shift-right: [w548] -> w545
                  shift-left: _ -> [w549]
                  tunnel: string[] ["STOP", "RESET ENCODERS", "RESET YAW", ""] -> [w547] mode=indexing
                  n216 = Enqueue Element(queue=w549, element=w547) -> (queue out=w548:refnum<queue>)  [unwired: 2 in, 2 out]
                }
              }
            }
          }
          frame 13 {
            w553 = u8 20
            # ">> Path blocked >>"
            # ">>> yStepper command>>>"
            # ">> Manual override >>"
            n217 = Dequeue Element(queue=w562, timeout in ms (-1)=w561, error in (no error)=w560) -> (element=w559:T7)  [unwired: 3 out]
            n218 = Less?(x=w555, y=w553) -> (x < y?=w550:bool)
            n219 = Less?(x=w554, y=w553) -> (x < y?=w551:bool)
            n220 = And(x=w551, y=w550) -> (x .and. y?=w552:bool)
            n221 = case shown="\"None\", Default" w559 {
              tunnel: [w576 State_Type_Definitions."True Stop" ("Enum")] -> w564
              tunnel: [w574 w591] -> w565
              tunnel: w558 -> [w573 _]
              tunnel: w563 -> [w567 _]
              tunnel: [State_Type_Definitions."Idle" ("Enum") State_Type_Definitions."Shutdown" ("Enum")] -> w557
              tunnel: w552 -> [w566 _]
              frame "None", Default {
                # ">> Manual override forces program to true stop >>"
                # ">>If ENABLE or Trigger is set to true>>"
                n222 = Or(x=w566, y=w567) -> (x .or. y?=w572:bool)
                n223 = case shown="False" w566 {
                  tunnel: [w579 w584] -> w574
                  tunnel: w573 -> [w578 w583]
                  frame False {
                    n224 = for {
                      shift-right: [w581] -> w579
                      shift-left: w578 -> [w582]
                      tunnel: string[] ["FORWARD", "READ ULTRASONIC", "READ YAW"] ("element") -> [w580] mode=indexing
                      n225 = Enqueue Element(queue=w582, element=w580) -> (queue out=w581:refnum<queue>)  [unwired: 2 in, 2 out]
                    }
                  }
                  frame True {
                    n226 = for {
                      shift-right: [w587] -> w584
                      shift-left: w583 -> [w588]
                      tunnel: string[] ["STOP", "RESET YAW", "RESET ENCODERS", "RESET FLAGS"] -> [w586] mode=indexing
                      n227 = Enqueue Element(queue=w588, element=w586) -> (queue out=w587:refnum<queue>)  [unwired: 2 in, 2 out]
                    }
                  }
                }
                n228 = Select(t=State_Type_Definitions."True Stop" ("Enum"), s=w567, f=State_Type_Definitions."Task 4_C" ("Enum")) -> (s? t:f=w569:T6)
                n229 = Select(t=w569, s=w572, f=State_Type_Definitions."Task 4_B" ("Enum")) -> (s? t:f=w576:T6)
              }
              frame "Exit" {
                n230 = for {
                  shift-right: [w594] -> w591
                  shift-left: _ -> [w595]
                  tunnel: string[] ["STOP", "RESET ENCODERS", "RESET YAW", ""] -> [w593] mode=indexing
                  n231 = Enqueue Element(queue=w595, element=w593) -> (queue out=w594:refnum<queue>)  [unwired: 2 in, 2 out]
                }
              }
            }
          }
          frame 14 {
            w605 = u8 20
            # ">> xDistance travelled>>"
            # ">> Path NOT blocked >>"
            # ">>> yStepper command>>>"
            # ">> Manual override >>"
            n232 = Dequeue Element(queue=w615, timeout in ms (-1)=w608, error in (no error)=w607) -> (element=w609:T7)  [unwired: 3 out]
            n233 = Greater?(x=w597, y=w605) -> (0:w603:bool)
            n234 = Greater?(x=w602, y=80.0) -> (0:w600:bool)
            n235 = Greater?(x=w596, y=w605) -> (0:w604:bool)
            n236 = And(x=w604, y=w603) -> (x .and. y?=w599:bool)
            n237 = And(x=w600, y=w599) -> (x .and. y?=w598:bool)
            n238 = case shown="\"None\", Default" w609 {
              tunnel: [w626 State_Type_Definitions."True Stop" ("Enum")] -> w612
              tunnel: [w624 w642] -> w611
              tunnel: w614 -> [w623 w639]
              tunnel: w613 -> [w617 _]
              tunnel: [State_Type_Definitions."Idle" ("t") State_Type_Definitions."Shutdown" ("Enum")] -> w610
              tunnel: w598 -> [w616 _]
              frame "None", Default {
                # ">> Manual override forces program to true stop >>"
                # ">>If ENABLE or Trigger is set to true>>"
                n239 = Or(x=w616, y=w617) -> (x .or. y?=w622:bool)
                n240 = case shown="True" w616 {
                  tunnel: [w629 w634] -> w624
                  tunnel: w623 -> [w627 w633]
                  frame False {
                    n241 = for {
                      shift-right: [w631] -> w629
                      shift-left: w627 -> [w632]
                      tunnel: string[] ["RIGHT", "READ YAW", "READ ENCODERS", "READ ULTRASONIC"] ("element") -> [w630] mode=indexing
                      n242 = Enqueue Element(queue=w632, element=w630) -> (queue out=w631:refnum<queue>)  [unwired: 2 in, 2 out]
                    }
                  }
                  frame True {
                    n243 = for {
                      shift-right: [w637] -> w634
                      shift-left: w633 -> [w638]
                      tunnel: string[] ["STOP", "RESET YAW", "RESET ENCODERS", "ARDUINO - ULTRASONIC"] -> [w636] mode=indexing
                      n244 = Enqueue Element(queue=w638, element=w636) -> (queue out=w637:refnum<queue>)  [unwired: 2 in, 2 out]
                    }
                  }
                }
                n245 = Select(t=State_Type_Definitions."True Stop" ("Enum"), s=w617, f=State_Type_Definitions."Task 4_D" ("Enum")) -> (s? t:f=w618:T6)
                n246 = Select(t=w618, s=w622, f=State_Type_Definitions."Task 4_C" ("Enum")) -> (s? t:f=w626:T6)
              }
              frame "Exit" {
                n247 = for {
                  shift-right: [w645] -> w642
                  shift-left: w639 -> [w646]
                  tunnel: string[] ["STOP", "RESET ENCODERS", "RESET YAW", ""] -> [w644] mode=indexing
                  n248 = Enqueue Element(queue=w646, element=w644) -> (queue out=w645:refnum<queue>)  [unwired: 2 in, 2 out]
                }
              }
            }
          }
          frame 15 {
            w665 = u8 20
            # ">> yDistance travelled>>"
            # ">> Path blocked >>"
            # ">>> yStepper command>>>"
            # ">> Manual override >>"
            n249 = Dequeue Element(queue=w656, timeout in ms (-1)=w655, error in (no error)=w654) -> (element=w666:T7)  [unwired: 3 out]
            n250 = Less?(x=w649, y=w665) -> (x < y?=w663:bool)
            n251 = Greater?(x=w653, y=200.0) -> (0:w661:bool)
            n252 = Less?(x=w648, y=w665) -> (x < y?=w664:bool)
            n253 = And(x=w664, y=w663) -> (x .and. y?=w660:bool)
            n254 = Or(x=w661, y=w660) -> (x .or. y?=w659:bool)
            n255 = case shown="\"None\", Default" w666 {
              tunnel: [w677 State_Type_Definitions."True Stop" ("Enum")] -> w652
              tunnel: [w675 w693] -> w650
              tunnel: w657 -> [w674 w690]
              tunnel: w658 -> [w668 _]
              tunnel: [State_Type_Definitions."Idle" ("t") State_Type_Definitions."Shutdown" ("Enum")] -> w651
              tunnel: w659 -> [w667 _]
              frame "None", Default {
                # ">> Manual override forces program to true stop >>"
                # ">>If ENABLE or Trigger is set to true>>"
                n256 = Or(x=w667, y=w668) -> (x .or. y?=w673:bool)
                n257 = case shown="False" w667 {
                  tunnel: [w680 w685] -> w675
                  tunnel: w674 -> [w678 w684]
                  frame False {
                    n258 = for {
                      shift-right: [w682] -> w680
                      shift-left: w678 -> [w683]
                      tunnel: string[] ["FORWARD", "READ YAW", "READ ENCODERS", "READ ULTRASONIC"] ("element") -> [w681] mode=indexing
                      n259 = Enqueue Element(queue=w683, element=w681) -> (queue out=w682:refnum<queue>)  [unwired: 2 in, 2 out]
                    }
                  }
                  frame True {
                    n260 = for {
                      shift-right: [w688] -> w685
                      shift-left: w684 -> [w689]
                      tunnel: string[] ["STOP", "RESET YAW", "RESET ENCODERS", "RESET FLAGS"] -> [w687] mode=indexing
                      n261 = Enqueue Element(queue=w689, element=w687) -> (queue out=w688:refnum<queue>)  [unwired: 2 in, 2 out]
                    }
                  }
                }
                n262 = Select(t=State_Type_Definitions."True Stop" ("Enum"), s=w668, f=State_Type_Definitions."True Stop" ("Enum")) -> (s? t:f=w669:T6)
                n263 = Select(t=w669, s=w673, f=State_Type_Definitions."Task 4_D" ("Enum")) -> (s? t:f=w677:T6)
              }
              frame "Exit" {
                n264 = for {
                  shift-right: [w696] -> w693
                  shift-left: w690 -> [w697]
                  tunnel: string[] ["STOP", "RESET ENCODERS", "RESET YAW", ""] -> [w695] mode=indexing
                  n265 = Enqueue Element(queue=w697, element=w695) -> (queue out=w696:refnum<queue>)  [unwired: 2 in, 2 out]
                }
              }
            }
          }
          frame 13 {
            # ">>> yStepper command>>>"
            # ">> Manual override >>"
            n266 = Dequeue Element(queue=w706, timeout in ms (-1)=w705, error in (no error)=w707) -> (element=w704:T7)  [unwired: 3 out]
            n267 = Equal?(x=w703, y=u8 80) -> (x = y?=w701:bool)
            n268 = case shown="\"None\", Default" w704 {
              tunnel: [w717 State_Type_Definitions."True Stop" ("Enum")] -> w708
              tunnel: [w720 w737] -> w709
              tunnel: [State_Type_Definitions."Idle" ("Enum") State_Type_Definitions."Shutdown" ("Enum")] -> w710
              tunnel: w701 -> [w716 _]
              tunnel: w700 -> [w715 _]
              tunnel: w699 -> [w711 w734]
              frame "None", Default {
                # "Stays in Task 5_A until stepper reaches desired \nheight"
                # "T: Go back to idle, F: Continue with task\""
                # ">> Manual override >>"
                n269 = case shown="True" w716 {
                  tunnel: [w724 w730] -> w720
                  tunnel: w711 -> [w722 w728]
                  frame False {
                    n270 = for {
                      tunnel: string[] ["Z STEPPER CAM HEIGHT", "READ STEPPER VALUES"] ("element") -> [w725] mode=indexing
                      shift-right: [w727] -> w724
                      shift-left: w722 -> [w726]
                      n271 = Enqueue Element(queue=w726, element=w725) -> (queue out=w727:refnum<queue>)  [unwired: 2 in, 2 out]
                    }
                  }
                  frame True {
                    n272 = for {
                      shift-right: [w732] -> w730
                      shift-left: w728 -> [w733]
                      tunnel: string[] ["ARDUINO - ULTRASONIC", "READ ULTRASONIC", ""] -> [w731] mode=indexing
                      n273 = Enqueue Element(queue=w733, element=w731) -> (queue out=w732:refnum<queue>)  [unwired: 2 in, 2 out]
                    }
                  }
                }
                n274 = Or(x=w716, y=w715) -> (x .or. y?=w718:bool)
                n275 = Select(t=State_Type_Definitions."True Stop" ("Enum"), s=w715, f=State_Type_Definitions."Task 5 _B" ("Enum")) -> (s? t:f=w712:u16)
                n276 = Select(t=w712, s=w718, f=State_Type_Definitions."Task 5_A" ("Enum")) -> (s? t:f=w717:u16)
              }
              frame "Exit" {
                n277 = for {
                  shift-right: [w740] -> w737
                  shift-left: w734 -> [w741]
                  tunnel: string[] ["STOP", "RESET ENCODERS", "RESET YAW", "ARDUINO MODE 0"] -> [w739] mode=indexing
                  n278 = Enqueue Element(queue=w741, element=w739) -> (queue out=w740:refnum<queue>)  [unwired: 2 in, 2 out]
                }
              }
            }
          }
          frame 14 {
            w747 = u8 20 ("y")
            # ">>> yStepper command>>>"
            n279 = Less?(x=w744, y=w747) -> (x < y?=w745:bool)
            n280 = Dequeue Element(queue=w751, timeout in ms (-1)=w750, error in (no error)=w752) -> (element=w749:T7)  [unwired: 3 out]
            n281 = Less?(x=w743, y=w747) -> (x < y?=w746:bool)
            n282 = And(x=w746, y=w745) -> (x .and. y?=w742:bool)
            n283 = case shown="\"None\", Default" w749 {
              tunnel: [w764 State_Type_Definitions."True Stop" ("Enum")] -> w754
              tunnel: [w767 w784] -> w753
              tunnel: [State_Type_Definitions."Idle" ("Enum") State_Type_Definitions."Shutdown" ("Enum")] -> w755
              tunnel: w757 -> [w763 _]
              tunnel: w756 -> [w759 w781]
              tunnel: w742 -> [w758 _]
              frame "None", Default {
                # "Stays in Task 5_B to capture image over 5 seconds"
                # "T: Go back to idle, F: Continue with task\""
                # ">> Manual override >>"
                n284 = case shown="True" w758 {
                  tunnel: [w771 w777] -> w767
                  tunnel: w759 -> [w769 w775]
                  frame False {
                    n285 = for {
                      tunnel: string[] ["FORWARD", "READ ULTRASONIC", "READ YAW"] ("element") -> [w772] mode=indexing
                      shift-right: [w774] -> w771
                      shift-left: w769 -> [w773]
                      n286 = Enqueue Element(queue=w773, element=w772) -> (queue out=w774:refnum<queue>)  [unwired: 2 in, 2 out]
                    }
                  }
                  frame True {
                    n287 = for {
                      shift-right: [w779] -> w777
                      shift-left: w775 -> [w780]
                      tunnel: string[] ["STOP", "RESET ENCODERS", "OPEN LOG CAM", "SET TIMER"] -> [w778] mode=indexing
                      n288 = Enqueue Element(queue=w780, element=w778) -> (queue out=w779:refnum<queue>)  [unwired: 2 in, 2 out]
                    }
                  }
                }
                n289 = Or(x=w758, y=w763) -> (x .or. y?=w765:bool)
                n290 = Select(t=State_Type_Definitions."True Stop" ("Enum"), s=w763, f=State_Type_Definitions."Task 5_C" ("Enum")) -> (s? t:f=w760:u16)
                n291 = Select(t=w760, s=w765, f=State_Type_Definitions."Task 5 _B" ("Enum")) -> (s? t:f=w764:u16)
              }
              frame "Exit" {
                n292 = for {
                  shift-right: [w787] -> w784
                  shift-left: w781 -> [w788]
                  tunnel: string[] ["STOP", "RESET ENCODERS", "RESET YAW", "ARDUINO MODE 0"] -> [w786] mode=indexing
                  n293 = Enqueue Element(queue=w788, element=w786) -> (queue out=w787:refnum<queue>)  [unwired: 2 in, 2 out]
                }
              }
            }
          }
          frame 15 {
            # ">>> yStepper command>>>"
            # ">> Manual override >>"
            n294 = Dequeue Element(queue=w797, timeout in ms (-1)=w796, error in (no error)=w795) -> (element=w794:T7)  [unwired: 3 out]
            n295 = case shown="\"None\", Default" w794 {
              tunnel: [w804 State_Type_Definitions."True Stop" ("Enum")] -> w799
              tunnel: [w807 w824] -> w792
              tunnel: [State_Type_Definitions."Idle" ("Enum") State_Type_Definitions."Shutdown" ("Enum")] -> w791
              tunnel: w793 -> [w801 _]
              tunnel: w798 -> [w803 w821]
              tunnel: w789 -> [w800 _]
              frame "None", Default {
                # ">> Is time up? >>"
                # "Determines if object is in range to pick up"
                # ">> Manual override >>"
                n296 = case shown="True" w800 {
                  tunnel: [w811 w817] -> w807
                  tunnel: w803 -> [w809 w815]
                  frame False {
                    n297 = for {
                      tunnel: string[] ["CAM ACQ", "START TIMER"] ("element") -> [w812] mode=indexing
                      shift-right: [w814] -> w811
                      shift-left: w809 -> [w813]
                      n298 = Enqueue Element(queue=w813, element=w812) -> (queue out=w814:refnum<queue>)  [unwired: 2 in, 2 out]
                    }
                  }
                  frame True {
                    n299 = for {
                      shift-right: [w819] -> w817
                      shift-left: w815 -> [w820]
                      tunnel: string[] ["CAM CLOSE", "PROCESS IMAGE"] -> [w818] mode=indexing
                      n300 = Enqueue Element(queue=w820, element=w818) -> (queue out=w819:refnum<queue>)  [unwired: 2 in, 2 out]
                    }
                  }
                }
                n301 = Or(x=w800, y=w801) -> (x .or. y?=w805:bool)
                n302 = Select(t=State_Type_Definitions."Task 5_D" ("Enum"), s=w805, f=State_Type_Definitions."Task 5_D" ("Enum")) -> (s? t:f=w804:T23)
              }
              frame "Exit" {
                n303 = for {
                  shift-right: [w827] -> w824
                  shift-left: w821 -> [w828]
                  tunnel: string[] ["STOP", "RESET ENCODERS", "RESET YAW", "ARDUINO MODE 0"] -> [w826] mode=indexing
                  n304 = Enqueue Element(queue=w828, element=w826) -> (queue out=w827:refnum<queue>)  [unwired: 2 in, 2 out]
                }
              }
            }
          }
          frame 16 {
            # ">>> yStepper command>>>"
            n305 = Dequeue Element(queue=w834, timeout in ms (-1)=w833, error in (no error)=w832) -> (element=w831:T7)  [unwired: 3 out]
            n306 = case shown="\"None\", Default" w831 {
              tunnel: [w846 State_Type_Definitions."True Stop" ("Enum")] -> w838
              tunnel: [w849 w866] -> w837
              tunnel: [State_Type_Definitions."Idle" ("Enum") State_Type_Definitions."Shutdown" ("Enum")] -> w839
              tunnel: w835 -> [w845 _]
              tunnel: w836 -> [w841 w863]
              tunnel: w829 -> [w840 _]
              frame "None", Default {
                # ">> T: Breaks out of state loop; F: Stays in loop>>"
                # ">> Manual override >>"
                # ">> Checks if object is detected>>"
                # "Stays in Task 5D until the object is detected"
                # "T: Go back to idle, F: Continue with task\""
                # ">> Manual override >>"
                n307 = case shown="True" w840 {
                  tunnel: [w853 w859] -> w849
                  tunnel: w841 -> [w851 w857]
                  frame False {
                    n308 = for {
                      tunnel: string[] ["PROCESS IMAGE", "", ""] ("element") -> [w854] mode=indexing
                      shift-right: [w856] -> w853
                      shift-left: w851 -> [w855]
                      n309 = Enqueue Element(queue=w855, element=w854) -> (queue out=w856:refnum<queue>)  [unwired: 2 in, 2 out]
                    }
                  }
                  frame True {
                    n310 = for {
                      shift-right: [w861] -> w859
                      shift-left: w857 -> [w862]
                      tunnel: string[] ["DISPOSE BUFFERS", "CAM CLOSE", ""] -> [w860] mode=indexing
                      n311 = Enqueue Element(queue=w862, element=w860) -> (queue out=w861:refnum<queue>)  [unwired: 2 in, 2 out]
                    }
                  }
                }
                n312 = Or(x=w840, y=w845) -> (x .or. y?=w847:bool)
                n313 = Select(t=State_Type_Definitions."True Stop" ("Enum"), s=w845, f=State_Type_Definitions."True Stop" ("Enum")) -> (s? t:f=w842:T6)
                n314 = Select(t=w842, s=w847, f=State_Type_Definitions."Task 5_D" ("Enum")) -> (s? t:f=w846:u16)
              }
              frame "Exit" {
                n315 = for {
                  shift-right: [w869] -> w866
                  shift-left: w863 -> [w870]
                  tunnel: string[] ["STOP", "RESET ENCODERS", "RESET YAW", "ARDUINO MODE 0"] -> [w868] mode=indexing
                  n316 = Enqueue Element(queue=w870, element=w868) -> (queue out=w869:refnum<queue>)  [unwired: 2 in, 2 out]
                }
              }
            }
          }
          frame 25 {
          }
          frame 25 {
            # ">>> yStepper command>>>"
            n317 = Dequeue Element(queue=w880, timeout in ms (-1)=w878, error in (no error)=w879) -> (element=w877:T7)  [unwired: 3 out]
            n318 = case shown="\"None\", Default" w877 {
              tunnel: [w887 State_Type_Definitions."True Stop" ("Enum")] -> w873
              tunnel: [w886 w905] -> w881
              tunnel: [State_Type_Definitions."Idle" ("Enum") State_Type_Definitions."Shutdown" ("Enum")] -> w874
              tunnel: w876 -> [w882 _]
              tunnel: w875 -> [w884 _]
              tunnel: w872 -> [w883 w902]
              frame "None", Default {
                # ">> Manual override >>"
                n319 = case shown="True" w884 {
                  tunnel: [w892 w898] -> w886
                  tunnel: w883 -> [w891 w896]
                  frame False {
                    n320 = for {
                      shift-right: [w895] -> w892
                      shift-left: w891 -> [w894]
                      tunnel: string[] ["CAM ACQ", "PROCESS IMAGE", "OPEN CLAW"] -> [w893] mode=indexing
                      n321 = Enqueue Element(queue=w894, element=w893) -> (queue out=w895:refnum<queue>)  [unwired: 2 in, 2 out]
                    }
                  }
                  frame True {
                    n322 = for {
                      shift-right: [w900] -> w898
                      shift-left: w896 -> [w901]
                      tunnel: string[] ["CAM ACQ", "PROCESS IMAGE", "CLOSE CLAW"] -> [w899] mode=indexing
                      n323 = Enqueue Element(queue=w901, element=w899) -> (queue out=w900:refnum<queue>)  [unwired: 2 in, 2 out]
                    }
                  }
                }
                n324 = Select(t=State_Type_Definitions."True Stop" ("Enum"), s=w882, f=State_Type_Definitions."Task 6_B" ("Enum")) -> (s? t:f=w887:T6)
              }
              frame "Exit" {
                # ">> State after true stop >>"
                # ">> Goes to true stop >>"
                n325 = for {
                  shift-right: [w908] -> w905
                  shift-left: w902 -> [w909]
                  tunnel: string[] ["STOP", "RESET ENCODERS", "RESET YAW", ""] -> [w907] mode=indexing
                  n326 = Enqueue Element(queue=w909, element=w907) -> (queue out=w908:refnum<queue>)  [unwired: 2 in, 2 out]
                }
              }
            }
          }
          frame 24 {
            # ">>> yStepper command>>>"
            n327 = Dequeue Element(queue=w917, timeout in ms (-1)=w916, error in (no error)=w915) -> (element=w922:T7)  [unwired: 3 out]
            n328 = Equal?(x=w913, y=u8 80) -> (x = y?=w912:bool)
            n329 = case shown="\"None\", Default" w922 {
              tunnel: [w929 State_Type_Definitions."True Stop" ("Enum")] -> w920
              tunnel: [w928 w946] -> w919
              tunnel: [State_Type_Definitions."Idle" ("Enum") State_Type_Definitions."Shutdown" ("Enum")] -> w921
              tunnel: w918 -> [w924 _]
              tunnel: w914 -> [w926 _]
              tunnel: w912 -> [w923 _]
              frame "None", Default {
                n330 = case shown="True" w923 {
                  tunnel: [w934 w940] -> w928
                  tunnel: w926 -> [w932 w938]
                  frame False {
                    n331 = for {
                      tunnel: string[] ["Z STEPPER CAM HEIGHT", "READ STEPPER VALUES"] ("element") -> [w935] mode=indexing
                      shift-right: [w937] -> w934
                      shift-left: w932 -> [w936]
                      n332 = Enqueue Element(queue=w936, element=w935) -> (queue out=w937:refnum<queue>)  [unwired: 2 in, 2 out]
                    }
                  }
                  frame True {
                    n333 = for {
                      shift-right: [w942] -> w940
                      shift-left: w938 -> [w943]
                      tunnel: string[] ["CAM ACQ", "OPEN LOG CAM"] -> [w941] mode=indexing
                      n334 = Enqueue Element(queue=w943, element=w941) -> (queue out=w942:refnum<queue>)  [unwired: 2 in, 2 out]
                    }
                  }
                }
                n335 = Or(x=w923, y=w924) -> (x .or. y?=w925:bool)
                n336 = Select(t=State_Type_Definitions."Task 6_B" ("Enum"), s=w925, f=State_Type_Definitions."Task 6_A" ("Enum")) -> (s? t:f=w929:T6)
              }
              frame "Exit" {
                n337 = for {
                  shift-right: [w949] -> w946
                  shift-left: _ -> [w950]
                  tunnel: string[] ["STOP", "RESET ENCODERS", "RESET YAW", "ARDUINO MODE 0"] -> [w948] mode=indexing
                  n338 = Enqueue Element(queue=w950, element=w948) -> (queue out=w949:refnum<queue>)  [unwired: 2 in, 2 out]
                }
              }
            }
          }
        }
      }
    }
    n339 = local write "Green LED"(w194) -> ()
  }
  n340 = call <vilib>:"DIO Close.vi"("error in (no error)"=w24, "DIO Info In"=w27) -> ()  [unwired: 9 in, 1 out]
  n341 = call <vilib>:"DIO Close.vi"("error in (no error)"=w34, "DIO Info In"=w36) -> ()  [unwired: 9 in, 1 out]
  n342 = call <vilib>:"NavX Close.vi"("error in (no error)"=w5, "NavX Info In"=w4) -> ()  [unwired: 9 in, 1 out]
  n343 = call <vilib>:"DIO Close.vi"("error in (no error)"=w29, "DIO Info In"=w31) -> ()  [unwired: 9 in, 1 out]
  n344 = call <vilib>:"DIO Close.vi"("error in (no error)"=w12, "DIO Info In"=w13) -> ()  [unwired: 9 in, 1 out]
  n345 = call <vilib>:"DIO Close.vi"("error in (no error)"=w7, "DIO Info In"=w8) -> ()  [unwired: 9 in, 1 out]
  n346 = while {
    stop <- w1383 stop-if-true
    n347 = call <vilib>:"RT Get CPU Loads.vi"() -> ("CPU loads"=→"CPU loads":T5[])  [unwired: 10 in, 1 out]
    n348 = Wait (ms)(milliseconds to wait=u32 100) -> ()  [unwired: 1 out]
    n349 = call "FGV Bool.vi"("Init/Read/Write State"=States_for_Action_Engine."Read") -> ("Output node"=w1383:bool)  [unwired: 2 in, 1 out]
  }
  n350 = while {
    stop <- w1387 stop-if-true
    n351 = call "MOTOR CONTROL WITH PID AE.vi"("AE Mode"=MOTOR_CONTROL_WITH_PID_AE_DATA_MODE_TYPE_DEF."Read from AE") -> ("Speed & distance"=→"Speed & distance":T1)  [unwired: 3 in]
    n352 = call "FGV Bool.vi"("Init/Read/Write State"=States_for_Action_Engine."Read") -> ("Output node"=w1387:bool)  [unwired: 2 in, 1 out]
    n353 = Wait (ms)(milliseconds to wait=u32 5) -> ()  [unwired: 1 out]
  }
  n354 = Merge Errors "Merge Errors"(w64, w63) -> (w46:errorcluster)
  n355 = Merge Errors(w50, w46) -> (w45:errorcluster)
  n356 = Destroy User Event(user event=w67, error in=w45) -> ()  [unwired: 1 out]
  n357 = Destroy User Event(user event=w68, error in=w45) -> ()  [unwired: 1 out]
  n358 = Unregister For Events(event registration refnum=w59, error in=w45) -> ()  [unwired: 1 out]
  n359 = Release Queue(queue=w41, error in (no error)=w45) -> (error out=w23:errorcluster)  [unwired: 1 in, 2 out]
  n360 = Release Queue(queue=w58, error in (no error)=w45) -> ()  [unwired: 1 in, 3 out]
  n361 = call <vilib>:"Simple Error Handler.vi"("error in (no error)"=w23) -> ("error out"=w22:errorcluster)  [unwired: 4 in, 4 out]
  n362 = call <vilib>:"Reset myRIO.vi"("error in (no error)"=w22) -> ("error out"=→"error out":errorcluster)  [unwired: 10 in]
